vi "Scan.vi"(7 "Cluster":T1, 8 "Error":refnum<vi>, 9 "EMERGENCY":refnum<vi>, 10 "Scan in Progress":refnum<vi>, 11 "QUIT":refnum<vi>) -> ()   [LabVIEW 2018]
uses:
  <vilib>/Utility/file.llb/Write To Spreadsheet File (string).vi
  <vilib>/Utility/file.llb/Read From Spreadsheet File (string).vi
panel:
  out "Set VB?":bool
  out "Set VA?":bool
  out "Set VB":refnum<vi>
  out "Set VA":refnum<vi>
  out "Voltage Supply A":refnum<vi>
  out "Voltage Supply B":refnum<vi>
  out "Total Actions":i32
  out "GM1 ULD":refnum<vi>
  out "GM2 ULD":refnum<vi>
  out "GM2 LLD":refnum<vi>
  out "GM1 LLD":refnum<vi>
  out "Observables":string[][](array[string])
  out "GM2 Dwell":refnum<vi>
  out "GM1 Dwell":refnum<vi>
  out "Measure GM2":refnum<vi>
  out "GM2 Counts":refnum<vi>
  out "Measure GM1":refnum<vi>
  out "GM1 Counts":refnum<vi>
  out "ABORT":bool
  out "6487 Samples/measurement":refnum<vi>
  out "6485 Samples/measurement":refnum<vi>
  out "Theta Go":refnum<vi>
  out "Run All":bool
  out "X (mm)":refnum<vi>
  out "Y (mm)":refnum<vi>
  out "Z (mm)":refnum<vi>
  out "Theta (deg)":refnum<vi>
  out "Keithley6485 Current (A)":refnum<vi>
  out "Keithley6487 Current (A)":refnum<vi>
  out "Measure 6487":refnum<vi>
  out "Measure 6485":refnum<vi>
  out "Motors Are Active":refnum<vi>
  out "Set Motors":refnum<vi>
  out "Set EG":refnum<vi>
  out "Keithley6487 Potential (V)":refnum<vi>
  out "EG Y2 Alignment (V)":refnum<vi>
  out "EG Y1 Alignment (V)":refnum<vi>
  out "EG X2 Alignment (V)":refnum<vi>
  out "EG X1 Alignment (V)":refnum<vi>
  out "EG Filament (V)":refnum<vi>
  out "EG Focus 2 (V)":refnum<vi>
  out "EG Focus 1 (V)":refnum<vi>
  out "EG Extraction (V)":refnum<vi>
  out "EG Energy (eV)":refnum<vi>
  out "EG Grid (V)":refnum<vi>
  out "Set EG?":bool
  out "Theta Go To (mm)":refnum<vi>
  out "Z Go":refnum<vi>
  out "Z Go To (mm)":refnum<vi>
  out "Y Go":refnum<vi>
  out "Y Go To (mm)":refnum<vi>
  out "X Go To (mm)":refnum<vi>
  out "X Go":refnum<vi>
  out "Set Motors?":bool
  out "Current Task":string[](array[string])
  in  "Tasks":string[][](array[string])
  out "Independent Variables":string[][](array[string])
  in  "Scan.vi":enum32{"Scan", "Settings"}(tab)
  in  "Load Scan":bool
  in  "Generate Scan":bool
  in  "Dummy":dbl
  in  "Stop Scan":bool
  out "Status":string
  in  "Start Counting From...":i32
  out "Current File":path
  in  "Pending Tasks":i32(listbox)
  in  "Delete Task":bool
  in  "Clear Queue":bool
  out "Current Scan":string
  out "Current Action":string caption="Next Action"
  in  "Run All Scans":bool
  in  "Run One Scan":bool
  in  "Measurements":i32[](listbox)=[0]
  in  "Add to Queue":bool
  in  "Step Size":dbl=2.0 min=0.0 format="%#_4g"
  in  "End":dbl=11.0 format="%#_4g"
  in  "Start":dbl=1.0 format="%#_4g"
  in  "Variable":u16(ring) items=["X (mm)", "Y (mm)", "Z (mm)", "Theta (deg)", "EG Grid (V)", "EG Energy (eV)", "EG Extraction (V)", "EG Focus 1 (V)", "EG Focus 2 (V)", "EG Filament (V)", "EG X1 Alignment (V)", "EG X2 Alignment (V)", "EG Y1 Alignment (V)", "EG Y2 Alignment (V)", "6485 Samples", "6487 Samples", "6487 Voltage (V)", "GM2 Dwell Time (s)", "GM2 SCA Lower Limit (V)", "GM2 SCA Upper Limit (V)", "GM1 Dwell Time (s)", "GM1 SCA Lower Limit (V)", "GM1 SCA Upper Limit (V)", "Voltage Supply A", "Voltage Supply B", "Dummy"]
  in  "Folder":path=path "C:/data" caption="Save Directory"
  in  "Output Filename":string="Scan"
  in  "Scan File":path=path "C:/LabView VIs/IPES Scan Generator/Complex_Scan.scan"
  out "Progress:":i32
  in  "Settling time (ms)":u32
  in  "Output File Extension":string="dat"
  in  "Spacer in Output Filenames":string="_"
  in  "Number of Digits in Output Filename Suffix":i32=2
  in  "Character That Separates Parameters in Scan Commands":string=";"
  out "Observables Old":string[](array[string])
  # "%"
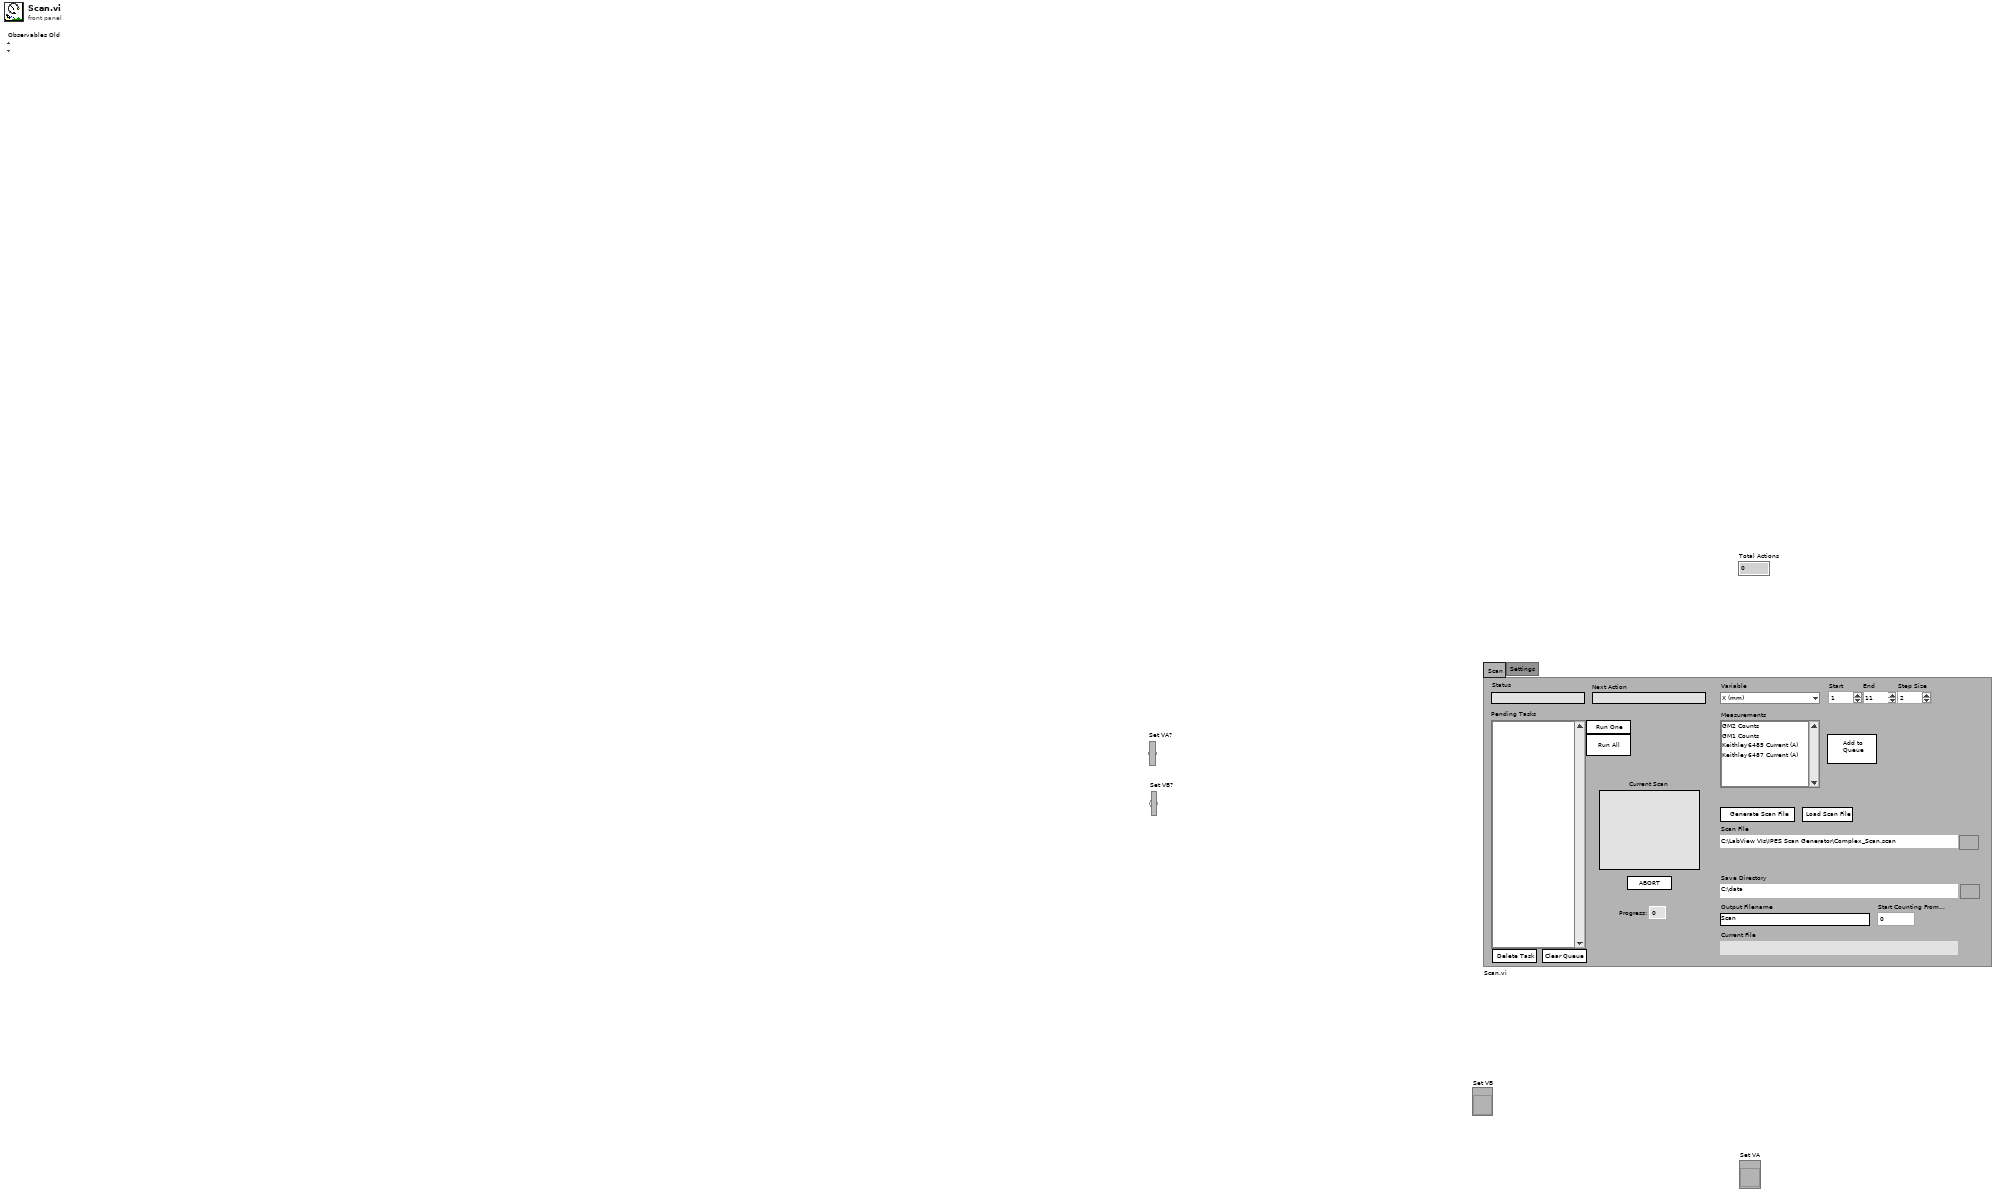
[diagram p1: front panel]
types:
  T1 = cluster{"EG Grid (V)":refnum<vi>, "EG Energy (eV)":refnum<vi>, "EG Extraction (V)":refnum<vi>, "EG Filament (V)":refnum<vi>, "EG Focus 1 (V)":refnum<vi>, "EG Focus 2 (V)":refnum<vi>, "EG X1 Alignment (V)":refnum<vi>, "EG X2 Alignment (V)":refnum<vi>, "EG Y1 Alignment (V)":refnum<vi>, "EG Y2 Alignment (V)":refnum<vi>, "Set EG":refnum<vi>, "X Go":refnum<vi>, "Y Go":refnum<vi>, "Z Go":refnum<vi>, "Theta Go":refnum<vi>, "X (mm)":refnum<vi>, "Y (mm)":refnum<vi>, "Z (mm)":refnum<vi>, "Theta (deg)":refnum<vi>, "X Go To (mm)":refnum<vi>, "Y Go To (mm)":refnum<vi>, "Z Go To (mm)":refnum<vi>, "Theta Go To (deg)":refnum<vi>, "Set Motors":refnum<vi>, "Motors Are Active":refnum<vi>, "Measure 6485":refnum<vi>, "Keithley6485 Current (A)":refnum<vi>, "6485 Samples/measurement":refnum<vi>, "Measure 6487":refnum<vi>, "Keithley6487 Current (A)":refnum<vi>, "Keithley6487 Voltage (V)":refnum<vi>, "6487 Samples/measurement":refnum<vi>, "GM Dwell Right":refnum<vi>, "GM LLD Right":refnum<vi>, "GM ULD Right":refnum<vi>, "GM Counts Right":refnum<vi>, "Measure GM Right":refnum<vi>, "GM Dwell Left":refnum<vi>, "GM LLD Left":refnum<vi>, "GM ULD Left":refnum<vi>, "GM Counts Left":refnum<vi>, "Measure GM Left":refnum<vi>, "Voltage Supply B":refnum<vi>, "Voltage Supply A":refnum<vi>, "Set VA":refnum<vi>, "Set VB":refnum<vi>}
  T2 = enum16{"open", "replace", "create", "open or create", "replace or create", "replace or create with confirmation"}
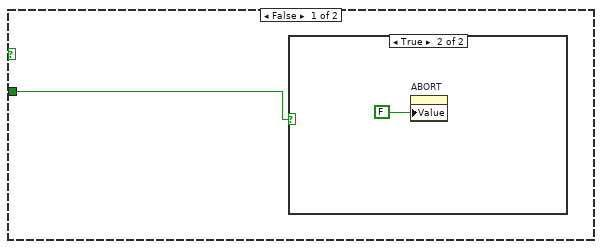
[diagram p14: hidden frame]
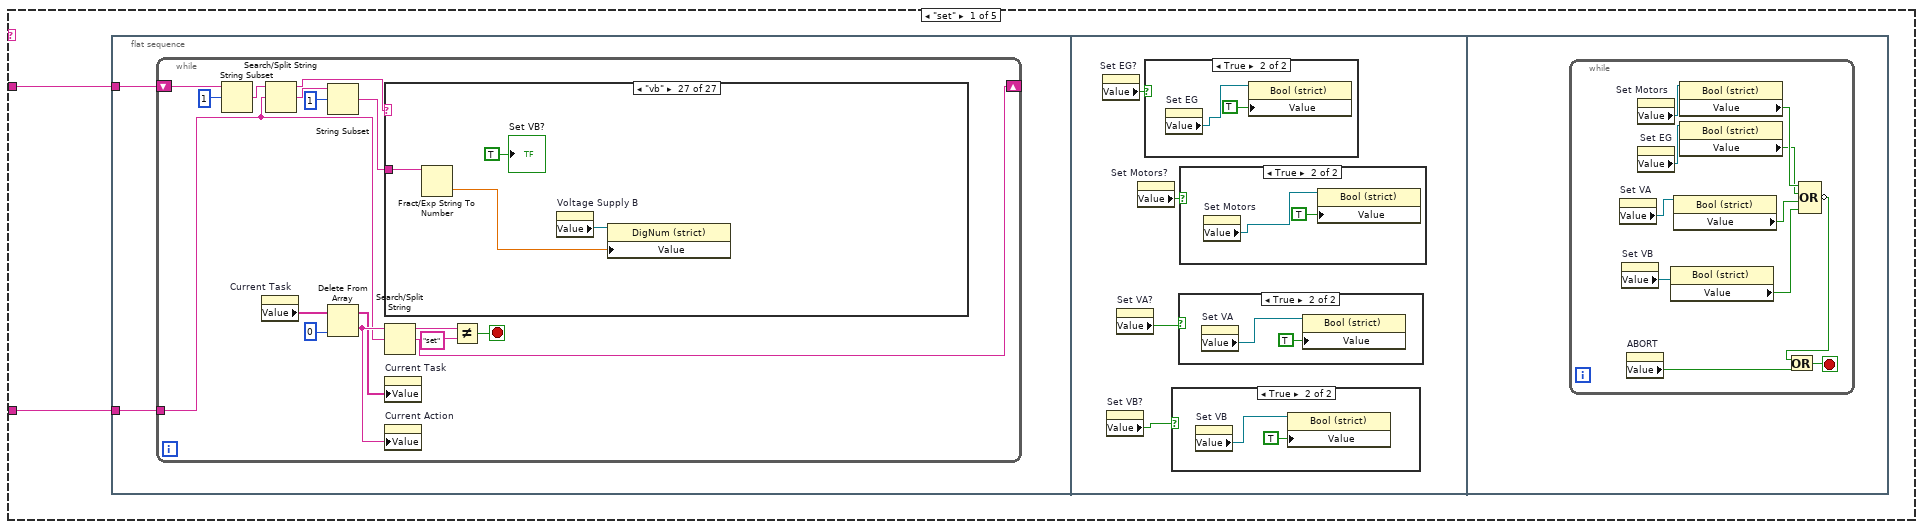
[diagram p17: hidden frame]
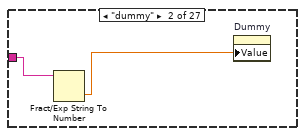
[diagram p19: hidden frame]
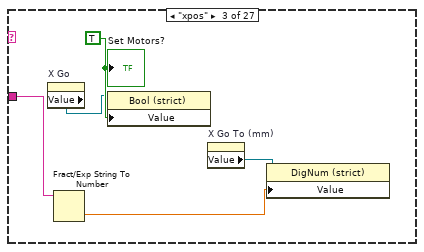
[diagram p20: hidden frame]
diagram:
  n1 = flat-sequence {
    frame #0 {
      w1 = FALSE ("Set Motors?")
      w2 = FALSE ("Visible")
      # "<Tasks> is a 2D list.  Every row represents a scan, and every element in a row is a scan command.  Note that rows can have different lengths.  When a scan is executed, it is popped off the top of <Tasks> and then its commands are executed in order.\n\n<Pending Tasks> is the 1D list of scans that the user sees.  Every element represents a scan and contains the meta data shown on the front panel."
      # "Initialization, variable declaration, etc..."
      n2 = Unbundle("Cluster") -> ("EG Grid (V)"=→"EG Grid (V)":refnum<vi>, "EG Energy (eV)"=→"EG Energy (eV)":refnum<vi>, "EG Extraction (V)"=→"EG Extraction (V)":refnum<vi>, "EG Filament (V)"=→"EG Filament (V)":refnum<vi>, "EG Focus 1 (V)"=→"EG Focus 1 (V)":refnum<vi>, "EG Focus 2 (V)"=→"EG Focus 2 (V)":refnum<vi>, "EG X1 Alignment (V)"=→"EG X1 Alignment (V)":refnum<vi>, "EG X2 Alignment (V)"=→"EG X2 Alignment (V)":refnum<vi>, "EG Y1 Alignment (V)"=→"EG Y1 Alignment (V)":refnum<vi>, "EG Y2 Alignment (V)"=→"EG Y2 Alignment (V)":refnum<vi>, "Set EG"=→"Set EG":refnum<vi>, "X Go"=→"X Go":refnum<vi>, "Y Go"=→"Y Go":refnum<vi>, "Z Go"=→"Z Go":refnum<vi>, "Theta Go"=→"Theta Go":refnum<vi>, "X (mm)"=→"X (mm)":refnum<vi>, "Y (mm)"=→"Y (mm)":refnum<vi>, "Z (mm)"=→"Z (mm)":refnum<vi>, "Theta (deg)"=→"Theta (deg)":refnum<vi>, "X Go To (mm)"=→"X Go To (mm)":refnum<vi>, "Y Go To (mm)"=→"Y Go To (mm)":refnum<vi>, "Z Go To (mm)"=→"Z Go To (mm)":refnum<vi>, "Theta Go To (deg)"=→"Theta Go To (mm)":refnum<vi>, "Set Motors"=→"Set Motors":refnum<vi>, "Motors Are Active"=→"Motors Are Active":refnum<vi>, "Measure 6485"=→"Measure 6485":refnum<vi>, "Keithley6485 Current (A)"=→"Keithley6485 Current (A)":refnum<vi>, "6485 Samples/measurement"=→"6485 Samples/measurement":refnum<vi>, "Measure 6487"=→"Measure 6487":refnum<vi>, "Keithley6487 Current (A)"=→"Keithley6487 Current (A)":refnum<vi>, "Keithley6487 Voltage (V)"=→"Keithley6487 Potential (V)":refnum<vi>, "6487 Samples/measurement"=→"6487 Samples/measurement":refnum<vi>, "GM Dwell Right"=→"GM1 Dwell":refnum<vi>, "GM LLD Right"=→"GM1 LLD":refnum<vi>, "GM ULD Right"=→"GM1 ULD":refnum<vi>, "GM Counts Right"=→"GM1 Counts":refnum<vi>, "Measure GM Right"=→"Measure GM1":refnum<vi>, "GM Dwell Left"=→"GM2 Dwell":refnum<vi>, "GM LLD Left"=→"GM2 LLD":refnum<vi>, "GM ULD Left"=→"GM2 ULD":refnum<vi>, "GM Counts Left"=→"GM2 Counts":refnum<vi>, "Measure GM Left"=→"Measure GM2":refnum<vi>, "Voltage Supply B"=→"Voltage Supply B":refnum<vi>, "Voltage Supply A"=→"Voltage Supply A":refnum<vi>, "Set VA"=→"Set VA":refnum<vi>, "Set VB"=→"Set VB":refnum<vi>)
      n3 = Initialize Array("", 0 ("dimension size")) -> (→"Current Task":string[])
      n4 = Build Array("gm2" ("element"), "gm1" ("element"), "6485c", "6487c") -> (w57:string[])
      n5 = Delete From Array(array="Tasks", index (col)=0 ("disabled index (col)")) -> (deleted portion=w117:string[])  [unwired: 2 in, 1 out]
      n6 = property on="Set VB?" class="Bool (strict)"("Value"=w1) -> ()  [unwired: 2 in, 2 out]
      n7 = property on="Set EG?" class="Bool (strict)"("Value"=w1) -> ()  [unwired: 2 in, 2 out]
      n8 = property on="Set Motors?" class="Bool (strict)"("Value"=w1) -> ()  [unwired: 2 in, 2 out]
      n9 = property on="Set VA?" class="Bool (strict)"("Value"=w1) -> ()  [unwired: 2 in, 2 out]
      n10 = property on="Pending Tasks" class="LstBox (strict)"("Item Names"=w117) -> ()  [unwired: 2 in, 2 out]
      n11 = Build Array("GM2 Counts" ("element"), "GM1 Counts" ("element"), "Keithley6485 Current (A)", "Keithley6487 Current (A)") -> (w58:string[])
      n12 = Build Array(w58, w57) -> (→"Observables":string[][])
      n13 = property on="Measurements" class="LstBox (strict)"("Item Names"=w58) -> ()  [unwired: 2 in, 2 out]
      n14 = Build Array("xpos", "ypos", "zpos", "theta", "grid", "en", "ext", "f1", "f2", "fil", "x1", "x2", "y1", "y2", "6485s", "6487s", "6487v", "gm2dw" ("element"), "gm2ll" ("element"), "gm2ul" ("element"), "gm1dw" ("element"), "gm1ll" ("element"), "gm1ul" ("element"), "va" ("element"), "vb" ("element"), "dummy" ("element")) -> (w116:string[])
      n15 = Build Array("X (mm)", "Y (mm)", "Z (mm)", "Theta (deg)", "EG Grid (V)", "EG Energy (eV)", "EG Extraction (V)", "EG Focus 1 (V)", "EG Focus 2 (V)", "EG Filament (V)", "EG X1 Alignment (V)", "EG X2 Alignment (V)", "EG Y1 Alignment (V)", "EG Y2 Alignment (V)", "6485 Samples", "6487 Samples", "6487 Voltage (V)", "GM2 Dwell Time (s)" ("element"), "GM2 SCA Lower Limit (V)" ("element"), "GM2 SCA Upper Limit (V)" ("element"), "GM1 Dwell Time (s)" ("element"), "GM1 SCA Lower Limit (V)" ("element"), "GM1 SCA Upper Limit (V)" ("element"), "Voltage Supply A (V)" ("element"), "Voltage Supply B (V)" ("element"), "Dummy" ("element")) -> (w59:string[])
      n16 = Build Array(w59, w116) -> (→"Independent Variables":string[][])
      n17 = property on="Variable" class="Ring (strict)"("Strings []"=w59) -> ()  [unwired: 2 in, 2 out]
      n18 = property on="Set Motors" class="LVObjRef (strict)"("Visible"=w2) -> ()  [unwired: 2 in, 2 out]
      n19 = property on="X Go To (mm)" class="LVObjRef (strict)"("Visible"=w2) -> ()  [unwired: 2 in, 2 out]
      n20 = property on="Set EG" class="LVObjRef (strict)"("Visible"=w2) -> ()  [unwired: 2 in, 2 out]
      n21 = property on="Z Go" class="LVObjRef (strict)"("Visible"=w2) -> ()  [unwired: 2 in, 2 out]
      n22 = property on="Y Go" class="LVObjRef (strict)"("Visible"=w2) -> ()  [unwired: 2 in, 2 out]
      n23 = property on="X Go" class="LVObjRef (strict)"("Visible"=w2) -> ()  [unwired: 2 in, 2 out]
      n24 = property on="Set Motors?" class="Bool (strict)"("Visible"=w2) -> ()  [unwired: 2 in, 2 out]
      n25 = property on="EG Grid (V)" class="LVObjRef (strict)"("Visible"=w2) -> ()  [unwired: 2 in, 2 out]
      n26 = property on="EG Focus 1 (V)" class="LVObjRef (strict)"("Visible"=w2) -> ()  [unwired: 2 in, 2 out]
      n27 = property on="EG Focus 2 (V)" class="LVObjRef (strict)"("Visible"=w2) -> ()  [unwired: 2 in, 2 out]
      n28 = property on="Z Go To (mm)" class="LVObjRef (strict)"("Visible"=w2) -> ()  [unwired: 2 in, 2 out]
      n29 = property on="QUIT" class="LVObjRef (strict)"("Visible"=w2) -> ()  [unwired: 2 in, 2 out]
      n30 = property on="Y Go To (mm)" class="LVObjRef (strict)"("Visible"=w2) -> ()  [unwired: 2 in, 2 out]
      n31 = property on="X (mm)" class="LVObjRef (strict)"("Visible"=w2) -> ()  [unwired: 2 in, 2 out]
      n32 = property on="ABORT" class="Bool (strict)"("Visible"=w2) -> ()  [unwired: 2 in, 2 out]
      n33 = property on="Theta (deg)" class="LVObjRef (strict)"("Visible"=w2) -> ()  [unwired: 2 in, 2 out]
      n34 = property on="Theta Go" class="LVObjRef (strict)"("Visible"=w2) -> ()  [unwired: 2 in, 2 out]
      n35 = property on="Run All" class="Bool (strict)"("Visible"=w2) -> ()  [unwired: 2 in, 2 out]
      n36 = property on="Z (mm)" class="LVObjRef (strict)"("Visible"=w2) -> ()  [unwired: 2 in, 2 out]
      n37 = property on="Y (mm)" class="LVObjRef (strict)"("Visible"=w2) -> ()  [unwired: 2 in, 2 out]
      n38 = property on="Set EG?" class="Bool (strict)"("Visible"=w2) -> ()  [unwired: 2 in, 2 out]
      n39 = property on="Error" class="LVObjRef (strict)"("Visible"=w2) -> ()  [unwired: 2 in, 2 out]
      n40 = property on="Measure 6487" class="LVObjRef (strict)"("Visible"=w2) -> ()  [unwired: 2 in, 2 out]
      n41 = property on="EMERGENCY" class="LVObjRef (strict)"("Visible"=w2) -> ()  [unwired: 2 in, 2 out]
      n42 = property on="Measure 6485" class="LVObjRef (strict)"("Visible"=w2) -> ()  [unwired: 2 in, 2 out]
      n43 = property on="Dummy" class="DigNum (strict)"("Visible"=w2) -> ()  [unwired: 2 in, 2 out]
      n44 = property on="Current Task" class="Arr (strict)"("Visible"=w2) -> ()  [unwired: 2 in, 2 out]
      n45 = property on="Tasks" class="Arr (strict)"("Visible"=w2) -> ()  [unwired: 2 in, 2 out]
      n46 = property on="EG Y2 Alignment (V)" class="LVObjRef (strict)"("Visible"=w2) -> ()  [unwired: 2 in, 2 out]
      n47 = property on="Keithley6487 Potential (V)" class="LVObjRef (strict)"("Visible"=w2) -> ()  [unwired: 2 in, 2 out]
      n48 = property on="EG Filament (V)" class="LVObjRef (strict)"("Visible"=w2) -> ()  [unwired: 2 in, 2 out]
      n49 = property on="Theta Go To (mm)" class="LVObjRef (strict)"("Visible"=w2) -> ()  [unwired: 2 in, 2 out]
      n50 = property on="Independent Variables" class="Arr (strict)"("Visible"=w2) -> ()  [unwired: 2 in, 2 out]
      n51 = property on="EG X1 Alignment (V)" class="LVObjRef (strict)"("Visible"=w2) -> ()  [unwired: 2 in, 2 out]
      n52 = property on="EG Extraction (V)" class="LVObjRef (strict)"("Visible"=w2) -> ()  [unwired: 2 in, 2 out]
      n53 = property on="EG X2 Alignment (V)" class="LVObjRef (strict)"("Visible"=w2) -> ()  [unwired: 2 in, 2 out]
      n54 = property on="EG Energy (eV)" class="LVObjRef (strict)"("Visible"=w2) -> ()  [unwired: 2 in, 2 out]
      n55 = property on="EG Y1 Alignment (V)" class="LVObjRef (strict)"("Visible"=w2) -> ()  [unwired: 2 in, 2 out]
      n56 = property on="Motors Are Active" class="LVObjRef (strict)"("Visible"=w2) -> ()  [unwired: 2 in, 2 out]
      n57 = property on="6485 Samples/measurement" class="LVObjRef (strict)"("Visible"=w2) -> ()  [unwired: 2 in, 2 out]
      n58 = property on="Keithley6485 Current (A)" class="LVObjRef (strict)"("Visible"=w2) -> ()  [unwired: 2 in, 2 out]
      n59 = property on="Keithley6487 Current (A)" class="LVObjRef (strict)"("Visible"=w2) -> ()  [unwired: 2 in, 2 out]
      n60 = property on="Scan in Progress" class="LVObjRef (strict)"("Visible"=w2) -> ()  [unwired: 2 in, 2 out]
      n61 = property on="GM1 Counts" class="LVObjRef (strict)"("Visible"=w2) -> ()  [unwired: 2 in, 2 out]
      n62 = property on="Measure GM1" class="LVObjRef (strict)"("Visible"=w2) -> ()  [unwired: 2 in, 2 out]
      n63 = property on="Measure GM2" class="LVObjRef (strict)"("Visible"=w2) -> ()  [unwired: 2 in, 2 out]
      n64 = property on="GM2 Counts" class="LVObjRef (strict)"("Visible"=w2) -> ()  [unwired: 2 in, 2 out]
      n65 = property on="EG Y2 Alignment (V)" class="LVObjRef (strict)"("Visible"=w2) -> ()  [unwired: 2 in, 2 out]
      n66 = property on="GM1 Dwell" class="LVObjRef (strict)"("Visible"=w2) -> ()  [unwired: 2 in, 2 out]
      n67 = property on="Voltage Supply A" class="LVObjRef (strict)"("Visible"=w2) -> ()  [unwired: 2 in, 2 out]
      n68 = property on="6487 Samples/measurement" class="LVObjRef (strict)"("Visible"=w2) -> ()  [unwired: 2 in, 2 out]
      n69 = property on="GM2 Dwell" class="LVObjRef (strict)"("Visible"=w2) -> ()  [unwired: 2 in, 2 out]
      n70 = property on="GM1 LLD" class="LVObjRef (strict)"("Visible"=w2) -> ()  [unwired: 2 in, 2 out]
      n71 = property on="GM2 LLD" class="LVObjRef (strict)"("Visible"=w2) -> ()  [unwired: 2 in, 2 out]
      n72 = property on="Observables" class="Arr (strict)"("Visible"=w2) -> ()  [unwired: 2 in, 2 out]
      n73 = property on="GM2 ULD" class="LVObjRef (strict)"("Visible"=w2) -> ()  [unwired: 2 in, 2 out]
      n74 = property on="GM1 ULD" class="LVObjRef (strict)"("Visible"=w2) -> ()  [unwired: 2 in, 2 out]
      n75 = property on="Voltage Supply B" class="LVObjRef (strict)"("Visible"=w2) -> ()  [unwired: 2 in, 2 out]
      n76 = property on="Cluster" class="Clust (strict)"("Visible"=w2) -> ()  [unwired: 2 in, 2 out]
      "ABORT" <- FALSE ("ABORT")
    }
    frame #1 {
      n77 = while {
        stop <- w131 stop-if-true
        # "This loops deals with all the buttons, etc., for the user interface.  Constantly checking to see if a button has been pushed.  If it has, execute some action."
        n78 = property class="Bool (strict)"(reference="EMERGENCY") -> ("Value"=w126:bool)  [unwired: 1 in, 2 out]
        n79 = case shown="True" "Add to Queue" {
          frame False {
          }
          frame True {
            w264 = "\r\n"
            w280 = "%#g" ("format string")
            # "Generate the 1D scan and add it to <Tasks> and <Pending Tasks>."
            n80 = property on="Character That Separates Parameters in Scan Commands" class="Str"() -> ("Value"=w266:string)  [unwired: 2 in, 2 out]
            n81 = Initialize Array("", 0 ("dimension size")) -> (w297:string[])
            n82 = Array Size(array="Measurements") -> (size(s)=w300:i32)
            n83 = for {
              N: w300 -> [_]
              tunnel: "Measurements" -> [w326]
              tunnel: w266 -> [w312]
              shift-right: [w322] -> w296
              shift-left: w297 -> [w325]
              shift-right: [w320] -> w277
              shift-left: "" -> [w321]
              i -> [w317]
              n84 = property on="Observables" class="Arr (strict)"() -> ("Value"=w315:string[][])  [unwired: 2 in, 2 out]
              n85 = Equal To 0?(x=w317) -> (x = 0?=w316:bool)
              n86 = Index Array(array=w326, index=w317) -> (element=w314:i32)
              n87 = case shown="False" w316 {
                tunnel: [", " _] -> w319
                frame False {
                }
                frame True {
                }
              }
              n88 = Index Array(array=w315, index (row)=1 ("disabled index (row)"), index (col)=w314) -> (element=w318:string)
              n89 = Concatenate Strings("measure", w312, w318, w312) -> (w323:string)
              n90 = Concatenate Strings(w321, w319, w318) -> (w320:string)
              n91 = Build Array (concatenate)(w325, w323) -> (w322:string[])
            }
            n92 = Subtract(x="End", y="Start") -> (x-y=w310:dbl)
            n93 = Greater?(x="Start", y="End") -> (0:w303:bool)
            n94 = case shown="True" w303 {
              tunnel: "Step Size" -> [w328 w330]
              tunnel: [w328 w329] -> w302
              frame False {
              }
              frame True {
                n95 = Negate(x=w330) -> (-x=w329:dbl)
              }
            }
            n96 = Divide(x=w310, y="Step Size") -> (x/y=w305:dbl)
            n97 = property on="Independent Variables" class="Arr (strict)"() -> ("Value"=w276:string[][])  [unwired: 2 in, 2 out]
            n98 = Absolute Value(x=w305) -> (abs(x)=w304:dbl)
            n99 = Increment(x=w304) -> (x+1=w311:dbl)
            n100 = Round Toward -Infinity(1:w311) -> (0:w270:dbl)
            n101 = Index Array(array=w276, index (row)=0 ("disabled index (col)"), index (col)="Variable") -> (element=w309:string)
            n102 = Index Array(array=w276, index (row)=1 ("disabled index (col)"), index (col)="Variable") -> (element=w301:string)
            n103 = Initialize Array("", 0 ("dimension size")) -> (w292:string[])
            n104 = Format Value(format string=w280, value (0)="Start") -> (output string=w286:string)  [unwired: 1 in]
            n105 = Format Value(format string=w280, value (0)="Step Size") -> (output string=w283:string)  [unwired: 1 in]
            n106 = Format Value(format string=w280, value (0)="End") -> (output string=w281:string)  [unwired: 1 in]
            n107 = for {
              N: w270 -> [_]
              tunnel: w302 -> [w339]
              tunnel: "Start" -> [w341]
              tunnel: w266 -> [w331]
              tunnel: w301 -> [w342]
              tunnel: w296 -> [w334]
              shift-right: [w333] -> w295
              shift-left: w292 -> [w332]
              i -> [w338]
              n108 = Multiply(x=w339, y=w338) -> (x*y=w340:dbl)
              n109 = Add(x=w341, y=w340) -> (x+y=w337:dbl)
              n110 = Number To Fractional String(number=w337) -> (F-format string=w336:string)  [unwired: 3 in]
              n111 = Concatenate Strings("set" ("string"), w331, w342, w331, w336, w331) -> (w335:string)
              n112 = Build Array (concatenate)(w332, w335, w334) -> (w333:string[])
            }
            n113 = property on="Pending Tasks" class="LstBox (strict)"() -> ("Item Names"=w274:string[])  [unwired: 2 in, 2 out]
            n114 = Number To Decimal String(number=w270) -> (decimal integer string=w269:string)  [unwired: 1 in]
            n115 = Concatenate Strings(w309, w264, "From ", w286, " To ", w281, " By ", w283, w264, "Measure " ("string"), w277, w264, w269, " points" ("string")) -> (w290:string)
            n116 = Build Array (concatenate)(w274, w290) -> (w273:string[])
            n117 = property on="Pending Tasks" class="LstBox (strict)"("Item Names"=w273) -> ()  [unwired: 2 in, 2 out]
            n118 = Concatenate Strings("end" ("element"), w266) -> (w265:string)
            n119 = Build Array (concatenate)(w290, w295, w265) -> (w291:string[])
            n120 = property on="Tasks" class="Arr (strict)"() -> ("Value"=w272:string[][])  [unwired: 2 in, 2 out]
            n121 = Build Array (concatenate)(w272, w291) -> (w271:string[][])
            n122 = property on="Tasks" class="Arr (strict)"("Value"=w271) -> ()  [unwired: 2 in, 2 out]
          }
        }
        n123 = case shown="True" "Stop Scan" {
          frame False {
          }
          frame True {
            # "Abort current scan and don't run the next one (if any are queued)."
            n124 = call <vilib>:"Beep.vi"("use system alert? (T)"=FALSE, "duration (msec)"=u32 300 ("frequency (Hz)"), "frequency (Hz)"=u32 250 ("duration (msec)")) -> ()  [unwired: 9 in]
            n125 = property on="Run All" class="Bool (strict)"("Value"=FALSE ("Run All")) -> ()  [unwired: 2 in, 2 out]
            n126 = property on="Current Action" class="Str"("Value"="") -> ()  [unwired: 2 in, 2 out]
            n127 = property on="ABORT" class="Bool (strict)"("Value"=TRUE ("ABORT")) -> ()  [unwired: 2 in, 2 out]
            n128 = property on="Current Scan" class="Str"() -> ("Value"=w246:string)  [unwired: 2 in, 2 out]
            n129 = Initialize Array("", 0 ("dimension size")) -> (w241:string[])
            n130 = property on="Current Task" class="Arr (strict)"("Value"=w241) -> ()  [unwired: 2 in, 2 out]
            n131 = Concatenate Strings("~Aborted~\n" ("string"), w246) -> (w244:string)
            n132 = property on="Scan in Progress" class="LVObjRef (strict)"() -> ("Value"=w249:refnum<vi>)  [unwired: 2 in, 2 out]
            n133 = property on="Current Scan" class="Str"("Value"=w244) -> ()  [unwired: 2 in, 2 out]
            n134 = property on="Status" class="Str"("Value"="Aborting Scan" ("Status")) -> ()  [unwired: 2 in, 2 out]
            n135 = property class="Bool (strict)"(reference=w249, "Value"=FALSE) -> ()  [unwired: 1 in, 2 out]
          }
        }
        n136 = case shown="True" "Clear Queue" {
          frame False {
          }
          frame True {
            # "Remove all scans from the list of scans."
            n137 = Initialize Array("", 0 ("dimension size"), 0 ("dimension size")) -> (w253:string[][])
            n138 = Initialize Array("", 0) -> (w252:string[])
            n139 = property on="Tasks" class="Arr (strict)"("Value"=w253) -> ()  [unwired: 2 in, 2 out]
            n140 = property on="Pending Tasks" class="LstBox (strict)"("Item Names"=w252) -> ()  [unwired: 2 in, 2 out]
          }
        }
        n141 = case shown="True" "Delete Task" {
          frame False {
          }
          frame True {
            # "Remove the selected scan from the list of scans."
            n142 = property on="Pending Tasks" class="LstBox (strict)"() -> ("Item Names"=w263:string[])  [unwired: 2 in, 2 out]
            n143 = property on="Tasks" class="Arr (strict)"() -> ("Value"=w260:string[][])  [unwired: 2 in, 2 out]
            n144 = Delete From Array(array=w263, index="Pending Tasks") -> (array with subset deleted=w262:string[])  [unwired: 1 in, 1 out]
            n145 = property on="Pending Tasks" class="LstBox (strict)"("Item Names"=w262) -> ()  [unwired: 2 in, 2 out]
            n146 = Delete From Array(array=w260, index (row)="Pending Tasks") -> (array with subset deleted=w259:string[][])  [unwired: 2 in, 1 out]
            n147 = property on="Tasks" class="Arr (strict)"("Value"=w259) -> ()  [unwired: 2 in, 2 out]
          }
        }
        n148 = case shown="True" w126 {
          frame False {
          }
          frame True {
            # "Stop all scans."
            n149 = property on="ABORT" class="Bool (strict)"("Value"=TRUE ("ABORT")) -> ()  [unwired: 2 in, 2 out]
          }
        }
        n150 = property on="QUIT" class="LVObjRef (strict)"() -> ("Value"=w132:refnum<vi>)  [unwired: 2 in, 2 out]
        n151 = property class="Bool (strict)"(reference=w132) -> ("Value"=w131:bool)  [unwired: 1 in, 2 out]
        n152 = case shown="True" "Generate Scan" {
          frame False {
          }
          frame True {
            w204 = "\"" ("string")
            # "Execute the external scan generating application using OS functions.  Collect various information from the <settings.conf> configuration file."
            n153 = Current VI's Path() -> (path=w211:path)
            n154 = Current VI's Path() -> (path=w192:path)
            n155 = Strip Path(path=w211) -> (stripped path=w207:path)  [unwired: 1 out]
            n156 = Strip Path(path=w192) -> (stripped path=w196:path)  [unwired: 1 out]
            n157 = Strip Path(path=w207) -> (stripped path=w206:path)  [unwired: 1 out]
            n158 = Strip Path(path=w196) -> (stripped path=w197:path)  [unwired: 1 out]
            n159 = Build Path(base path=w206, name or relative path="IPES Scan Generator") -> (appended path=w209:path)
            n160 = Build Path(base path=w197, name or relative path="IPES Scan Generator") -> (appended path=w194:path)
            n161 = Path To String(path=w209) -> (string=w208:string)
            n162 = Path To String(path=w194) -> (string=w195:string)
            n163 = Concatenate Strings(w195, "\\src\\settings.conf" ("string")) -> (w191:string)
            n164 = String To Path(string=w191) -> (path=w190:path)
            n165 = Concatenate Strings("C:\\Python32\\python.exe " ("command line"), w204, w208, "/src/jener8or.py" ("string"), w204) -> (w202:string)
            n166 = Read from Text File(file (use dialog)=w190) -> (text=w175:string)  [unwired: 3 in, 3 out]
            n167 = while {
              tunnel: [w232] -> w200 mode=indexing
              tunnel: "[Pp][Aa][Tt][Hh][\\s\\t]+=[\\s\\t]+" ("search string") -> [w230]
              shift-right: [w229] -> _
              shift-left: w175 -> [w231]
              stop <- w228 stop-if-true
              n168 = Match Pattern(string=w231, regular expression=w230) -> (after substring=w233:string)  [unwired: 1 in, 3 out]
              n169 = Match Pattern(string=w233, regular expression="[\\n]") -> (before substring=w232:string, after substring=w229:string)  [unwired: 1 in, 2 out]
              n170 = Equal?(x=w232, y="") -> (x = y?=w228:bool)
            }
            n171 = call <vilib>:"System Exec.vi"("wait until completion? (T)"=FALSE, "command line"=w202) -> ()  [unwired: 6 in, 4 out]
            n172 = while {
              tunnel: [w224] -> w182 mode=indexing
              tunnel: "[Ff][Ii][Ll][Ee][Nn][Aa][Mm][Ee][\\s\\t]+=[\\s\\t]+" ("search string") -> [w222]
              shift-right: [w221] -> _
              shift-left: w175 -> [w223]
              stop <- w220 stop-if-true
              n173 = Match Pattern(string=w223, regular expression=w222) -> (after substring=w225:string)  [unwired: 1 in, 3 out]
              n174 = Match Pattern(string=w225, regular expression="[\\n]") -> (before substring=w224:string, after substring=w221:string)  [unwired: 1 in, 2 out]
              n175 = Equal?(x=w224, y="") -> (x = y?=w220:bool)
            }
            n176 = while {
              tunnel: [w216] -> w179 mode=indexing
              tunnel: "[Ss][Ee][Pp][Aa][Rr][Aa][Tt][Oo][Rr][\\s\\t]+=[\\s\\t\\]+" ("search string") -> [w214]
              shift-right: [w213] -> _
              shift-left: w175 -> [w215]
              stop <- w212 stop-if-true
              n177 = Match Pattern(string=w215, regular expression=w214) -> (after substring=w217:string)  [unwired: 1 in, 3 out]
              n178 = Match Pattern(string=w217, regular expression="[\\n]") -> (before substring=w216:string, after substring=w213:string)  [unwired: 1 in, 2 out]
              n179 = Equal?(x=w216, y="") -> (x = y?=w212:bool)
            }
            n180 = Array Size(array=w200) -> (size(s)=w199:i32)
            n181 = Array Size(array=w182) -> (size(s)=w183:i32)
            n182 = Array Size(array=w179) -> (size(s)=w176:i32)
            n183 = Decrement(x=w199) -> (x-1=w188:i32)
            n184 = Decrement(x=w183) -> (x-1=w184:i32)
            n185 = Decrement(x=w176) -> (x-1=w177:i32)
            n186 = Decrement(x=w188) -> (x-1=w187:i32)
            n187 = Decrement(x=w184) -> (x-1=w185:i32)
            n188 = Decrement(x=w177) -> (x-1=w178:i32)
            n189 = Index Array(array=w200, index=w187) -> (element=w173:string)
            n190 = Index Array(array=w182, index=w185) -> ()  [unwired: 1 out]
            n191 = Index Array(array=w179, index=w178) -> (element=w181:string)
            n192 = property on="Character That Separates Parameters in Scan Commands" class="Str"("Value"=w181) -> ()  [unwired: 2 in, 2 out]
            n193 = String To Path(string=w173) -> (path=w174:path)
            n194 = property on="Scan File" class="Path"("Value"=w174) -> ()  [unwired: 2 in, 2 out]
          }
        }
        n195 = Or(x="Run One Scan", y="Run All Scans") -> (x .or. y?=w125:bool)
        n196 = case shown="True" w125 {
          tunnel: "Run All Scans" -> [_ w357]
          frame False {
          }
          frame True {
            # "Toggle the <Scan in Progress> flag on.  Turn all <Set #> and <Measure #> flags off.  If the user pressed \"Run All Scans,\" then turn the <Run All> flag on."
            n197 = property on="Run All" class="Bool (strict)"("Value"=w357) -> ()  [unwired: 2 in, 2 out]
            n198 = property on="Scan in Progress" class="LVObjRef (strict)"() -> ("Value"=w359:refnum<vi>)  [unwired: 2 in, 2 out]
            n199 = property class="Bool (strict)"(reference=w359, "Value"=TRUE ("Scan In Progress")) -> ()  [unwired: 1 in, 2 out]
            n200 = property on="Status" class="Str"("Value"="Initializing Scan\n(Getting Last Measurements)") -> ()  [unwired: 2 in, 2 out]
            n201 = property on="Set EG" class="LVObjRef (strict)"() -> ("Value"=w354:refnum<vi>)  [unwired: 2 in, 2 out]
            n202 = property on="Set Motors" class="LVObjRef (strict)"() -> ("Value"=w355:refnum<vi>)  [unwired: 2 in, 2 out]
            n203 = property class="Bool (strict)"(reference=w354, "Value"=FALSE) -> ()  [unwired: 1 in, 2 out]
            n204 = property class="Bool (strict)"(reference=w355, "Value"=FALSE) -> ()  [unwired: 1 in, 2 out]
            n205 = disable-structure shown="Disabled" {
              frame Disabled {
                n206 = property on="Measure GM2" class="LVObjRef (strict)"() -> ("Value"=w360:refnum<vi>)  [unwired: 2 in, 2 out]
                n207 = property class="Bool (strict)"(reference=w360, "Value"=TRUE) -> ()  [unwired: 1 in, 2 out]
              }
              frame Enabled {
              }
            }
            n208 = property on="Measure GM1" class="LVObjRef (strict)"() -> ("Value"=w351:refnum<vi>)  [unwired: 2 in, 2 out]
            n209 = property class="Bool (strict)"(reference=w351, "Value"=TRUE) -> ()  [unwired: 1 in, 2 out]
            n210 = property on="Measure 6485" class="LVObjRef (strict)"() -> ("Value"=w349:refnum<vi>)  [unwired: 2 in, 2 out]
            n211 = property on="Measure 6487" class="LVObjRef (strict)"() -> ("Value"=w346:refnum<vi>)  [unwired: 2 in, 2 out]
            n212 = property class="Bool (strict)"(reference=w349, "Value"=TRUE ("Measure 6485")) -> ()  [unwired: 1 in, 2 out]
            n213 = property class="Bool (strict)"(reference=w346, "Value"=TRUE ("Measure 6485")) -> ()  [unwired: 1 in, 2 out]
            n214 = property on="Set EG?" class="Bool (strict)"("Value"=FALSE ("Set EG?")) -> ()  [unwired: 2 in, 2 out]
            n215 = property on="Set Motors?" class="Bool (strict)"("Value"=FALSE ("Set Motors?")) -> ()  [unwired: 2 in, 2 out]
          }
        }
        n216 = case shown="True" "Load Scan" {
          frame False {
          }
          frame True {
            # "Load a scan from the specified file and add it to <Tasks>.  Add meta data to <Pending Tasks>."
            n217 = call-poly <vilib>:"Read From Spreadsheet File.vi"("file path (dialog if empty)"="Scan File") -> ("all rows"=w153:string[][])  [unwired: 6 in, 4 out]
            n218 = Index Array(array=w153, index (col)=0 ("disabled index (col)")) -> (element=w149:string[])  [unwired: 1 in]
            n219 = while {
              shift-right: [w158] -> _
              shift-left: w149 -> [w160]
              tunnel: [w159] -> w147 mode=indexing
              tunnel: [w158] -> w138
              stop <- w162 continue-if-true
              n220 = Delete From Array(array=w160, index=0) -> (deleted portion=w163:string, array with subset deleted=w161:string[])  [unwired: 1 in]
              n221 = String Subset(string=w163, length (rest)=1 ("length (rest)")) -> (substring=w165:string)  [unwired: 1 in]
              n222 = Equal?(x="#" ("search string"), y=w165) -> (x = y?=w162:bool)
              n223 = case shown="True" w162 {
                tunnel: w163 -> [_ w172]
                tunnel: [_ w170] -> w159
                tunnel: [w168 w169] -> w158
                tunnel: w161 -> [_ w169]
                tunnel: w160 -> [w168 _]
                frame False {
                }
                frame True {
                  n224 = String Subset(string=w172, offset (0)=1) -> (substring=w170:string)  [unwired: 1 in]
                }
              }
            }
            n225 = Array Size(array=w147) -> (size(s)=w148:i32)
            n226 = for {
              N: w148 -> [_]
              tunnel: w147 -> [w156] mode=indexing
              shift-right: [w155] -> w143
              shift-left: "" -> [w157]
              n227 = Concatenate Strings(w157, w156, "\r\n") -> (w155:string)
            }
            n228 = String Length(string=w143) -> (length=w142:i32)
            n229 = property on="Pending Tasks" class="LstBox (strict)"() -> ("Item Names"=w145:string[])  [unwired: 2 in, 2 out]
            n230 = Subtract(x=w142, y=4) -> (x-y=w141:i32)
            n231 = String Subset(string=w143, length (rest)=w141) -> (substring=w137:string)  [unwired: 1 in]
            n232 = property on="Tasks" class="Arr (strict)"() -> ("Value"=w151:string[][])  [unwired: 2 in, 2 out]
            n233 = Build Array (concatenate)(w137, w138) -> (w139:string[])
            n234 = Build Array (concatenate)(w145, w137) -> (w144:string[])
            n235 = Build Array (concatenate)(w151, w139) -> (w150:string[][])
            n236 = property on="Pending Tasks" class="LstBox (strict)"("Item Names"=w144) -> ()  [unwired: 2 in, 2 out]
            n237 = property on="Tasks" class="Arr (strict)"("Value"=w150) -> ()  [unwired: 2 in, 2 out]
          }
        }
      }
      n238 = while {
        stop <- w369 stop-if-true
        # "This loop handles the actual scanning algorithm."
        n239 = property on="QUIT" class="LVObjRef (strict)"() -> ("Value"=w368:refnum<vi>)  [unwired: 2 in, 2 out]
        n240 = property class="Bool (strict)"(reference=w368) -> ("Value"=w369:bool)  [unwired: 1 in, 2 out]
        n241 = property on="EMERGENCY" class="LVObjRef (strict)"() -> ("Value"=w364:refnum<vi>)  [unwired: 2 in, 2 out]
        n242 = property class="Bool (strict)"(reference=w364) -> ("Value"=w366:bool)  [unwired: 1 in, 2 out]
        n243 = property on="Scan in Progress" class="LVObjRef (strict)"() -> ("Value"=w365:refnum<vi>)  [unwired: 2 in, 2 out]
        n244 = property class="Bool (strict)"(reference=w365) -> ("Value"=w363:bool)  [unwired: 1 in, 2 out]
        n245 = Not(x=w366) -> (.not. x?=w362:bool)
        n246 = And(x=w363, y=w362) -> (x .and. y?=w367:bool)
        n247 = case shown="True" w367 {
          tunnel: w362 -> [w370 _]
          frame False {
            n248 = case shown="True" w370 {
              frame False {
              }
              frame True {
                n249 = property on="ABORT" class="Bool (strict)"("Value"=FALSE ("ABORT")) -> ()  [unwired: 2 in, 2 out]
              }
            }
          }
          frame True {
            # "Enter this structure if there's a scan running and no emergency."
            n250 = property on="Tasks" class="Arr (strict)"() -> ("Value"=w372:string[][])  [unwired: 2 in, 2 out]
            n251 = property on="Current Task" class="Arr (strict)"() -> ("Value"=w373:string[])  [unwired: 2 in, 2 out]
            n252 = Array Size(array=w372) -> (size(s)=w378:i32[])
            n253 = Array Size(array=w373) -> (size(s)=w376:i32)
            n254 = Index Array(array=w378, index=0) -> (element=w379:i32)
            n255 = Equal To 0?(x=w379) -> (x = 0?=w375:bool)
            n256 = Equal To 0?(x=w376) -> (x = 0?=w374:bool)
            n257 = And(x=w375, y=w374) -> (x .and. y?=w377:bool)
            n258 = case shown="False" w377 {
              tunnel: w374 -> [w382 _]
              tunnel: w373 -> [w381 _]
              frame False {
                # "Enter this structure if NOT (<Current Task> is empty AND <Tasks> is empty).  i.e. <Current Task> or <Tasks> has at least one element left to execute."
                n259 = flat-sequence {
                  tunnel: w382 -> [w402]
                  tunnel: w381 -> [w401]
                  frame #0 {
                    # "Pop the top element off <Current Task> and write it to <Current Action> for display to the user."
                    n260 = case shown="True" w402 {
                      tunnel: [w726 w730] -> w393
                      tunnel: w401 -> [w726 _]
                      frame False {
                      }
                      frame True {
                        w750 = "#" ("string")
                        w760 = "#" ("string")
                        w758 = "\r\n"
                        # "Order of execution:\n-Pop the top row off of <Tasks> and set it to <Current Task>.\n-Overwrite <Pending Tasks> with the first column of <Tasks>.\n-Pop the first element off of <Current Tasks> (should contain meta data) and display it to the user in <Current Scan>.\n-Use the \"File Name Gen\" subVI to calculate the output data file name.\n-Generate the header for the output file using the filename, the current time, and the meta data in <Current Scan>.\n-Open the file, write the header, then close the file.\n-Generate the first 2 columns of \"data\" (really, it's more header).  The first column is the long names of the independent variables and observables.  The second column is the short names.  Note that a \"#\" is added to the beginning of each column to indicate that it's a header.\n-Write the first 2 columns to the file using the \"Write to Spreadsheet File\" subVI.\n-Output <Current Task> from the structure, with blank entries removed."
                        # "Enter this structure if <Current Task> is empty."
                        # "Make new file"
                        # "Make file header"
                        n261 = property on="Tasks" class="Arr (strict)"() -> ("Value"=w736:string[][])  [unwired: 2 in, 2 out]
                        n262 = Delete From Array(array=w736, index (row)=0) -> (deleted portion=w770:string[], array with subset deleted=w772:string[][])  [unwired: 2 in]
                        n263 = property on="Tasks" class="Arr (strict)"("Value"=w772) -> ()  [unwired: 2 in, 2 out]
                        n264 = property on="Current Task" class="Arr (strict)"("Value"=w770) -> ()  [unwired: 2 in, 2 out]
                        n265 = Concatenate Strings(w758, w760) -> (w757:string)
                        n266 = Delete From Array(array=w772, index (col)=0 ("disabled index (col)")) -> (deleted portion=w771:string[])  [unwired: 2 in, 1 out]
                        n267 = Delete From Array(array=w770, index=0) -> (deleted portion=w761:string, array with subset deleted=w735:string[])  [unwired: 1 in]
                        "Current Scan" <- w761
                        n268 = property on="Pending Tasks" class="LstBox (strict)"("Item Names"=w771) -> ()  [unwired: 2 in, 2 out]
                        n269 = Search and Replace String(replace all?=TRUE ("replace all? (F)"), input string=w761, search string=w758, replace string=w757) -> (result string=w756:string)  [unwired: 4 in, 3 out]
                        n270 = call "filename generator (number).vi"("create folder?"=TRUE, "digits (2)"="Number of Digits in Output Filename Suffix", "separator (none)"="Spacer in Output Filenames", "start number (0)"="Start Counting From...", "extension"="Output File Extension", "filename root"="Output Filename", "root folder"="Folder") -> ("filename"=w773:path)  [unwired: 3 in, 1 out]
                        "Current File" <- w773
                        n271 = Array Size(array=w735) -> (size(s)=w734:i32)
                        n272 = Strip Path(path=w773) -> (name=w783:string)  [unwired: 1 out]
                        n273 = Initialize Array("" ("element"), 0 ("dimension size")) -> (w731:string[])
                        n274 = Get Date/Time String(want seconds? (F)=TRUE) -> (date string=w781:string, time string=w779:string)  [unwired: 2 in]
                        n275 = for {
                          N: w734 -> [_]
                          tunnel: w735 -> [w802]
                          shift-right: [w797] -> w730
                          shift-left: w731 -> [w801]
                          i -> [w803]
                          n276 = Index Array(array=w802, index=w803) -> (element=w796:string)
                          n277 = property on="Character That Separates Parameters in Scan Commands" class="Str"() -> ("Value"=w804:string)  [unwired: 2 in, 2 out]
                          n278 = Search/Split String(string=w796, search string/char (-)=w804) -> (substring before match=w800:string)  [unwired: 1 in, 2 out]
                          n279 = Equal?(x="" ("element"), y=w800) -> (x = y?=w798:bool)
                          n280 = case shown="False" w798 {
                            tunnel: w801 -> [w807 w808]
                            tunnel: [w806 w808] -> w797
                            tunnel: w796 -> [w805 _]
                            frame False {
                              n281 = Build Array (concatenate)(w807, w805) -> (w806:string[])
                            }
                            frame True {
                            }
                          }
                        }
                        n282 = call <vilib>:"Space Constant.vi"() -> ("String"=w780:string)
                        n283 = property on="Error" class="LVObjRef (strict)"() -> ("Value"=w764:refnum<vi>)  [unwired: 2 in, 2 out]
                        n284 = Concatenate Strings(w760, w783, w758, w760, w781, w780, w779, w758, w760, w756, w758) -> (w778:string)
                        n285 = property class="Clust (strict)"(reference=w764) -> (reference out=w765:refnum<vi>, "Value"=w767:errorcluster)  [unwired: 1 in, 1 out]
                        n286 = property on="Independent Variables" class="Arr (strict)"() -> ("Value"=w752:string[][])  [unwired: 2 in, 2 out]
                        n287 = property on="Observables" class="Arr (strict)"() -> ("Value"=w745:string[][])  [unwired: 2 in, 2 out]
                        n288 = Open/Create/Replace File(file path (use dialog)=w773, error in=w767, operation (0:open)=T2."create") -> (refnum out=w789:refnum<file>, error out=w788:errorcluster)  [unwired: 3 in, 1 out]
                        n289 = Write to Text File(file (use dialog)=w789, text=w778, error in=w788) -> (refnum out=w787:refnum<file>, error out=w786:errorcluster)  [unwired: 1 in, 1 out]
                        n290 = Delete From Array(array=w752, index (row)=0) -> (deleted portion=w737:string[])  [unwired: 2 in, 1 out]
                        n291 = Index Array(array=w745, index (row)=0) -> (element=w762:string[])  [unwired: 1 in]
                        n292 = Delete From Array(array=w752, index (row)=1) -> (deleted portion=w738:string[])  [unwired: 2 in, 1 out]
                        n293 = Index Array(array=w745, index (row)=1) -> (element=w743:string[])  [unwired: 1 in]
                        n294 = Close File(refnum=w787, error in=w786) -> (path=w795:path, error out=w766:errorcluster)
                        n295 = property class="Clust (strict)"(reference=w765, "Value"=w766) -> ()  [unwired: 1 in, 2 out]
                        n296 = Concatenate Strings(w750, "time") -> (w749:string)
                        n297 = Concatenate Strings(w750, "Timestamp (sec)") -> (w755:string)
                        n298 = Array Size(array=w730) -> (size(s)=w729:i32)
                        n299 = Insert Into Array(array=w737, index=0, new element=w755) -> (w753:string[])
                        n300 = Insert Into Array(array=w753, new element=w762) -> (w747:string[])  [unwired: 1 in]
                        n301 = Insert Into Array(array=w738, index=0, new element=w749) -> (w742:string[])
                        n302 = Subtract(x=w729, y=1) -> (x-y=→"Total Actions":i32)
                        n303 = Insert Into Array(array=w742, new element=w743) -> (w741:string[])  [unwired: 1 in]
                        n304 = Build Array(w747, w741) -> (w746:string[][])
                        n305 = call-poly <vilib>:"Write To Spreadsheet File.vi"("append to file? (new file:F)"=TRUE, "2D data"=w746, "file path (dialog if empty)"=w795) -> ()  [unwired: 5 in, 1 out]
                      }
                    }
                    n306 = property on="Status" class="Str"("Value"="Scanning" ("Status")) -> ()  [unwired: 2 in, 2 out]
                    n307 = Array Size(array=w393) -> (size(s)=w392:i32)
                    n308 = property on="Total Actions" class="DigNum (strict)"() -> ("Value"=w391:i32)  [unwired: 2 in, 2 out]
                    n309 = Divide(x=w392, y=w391) -> (x/y=w389:dbl)
                    n310 = Subtract(x=1, y=w389) -> (x-y=w387:dbl)
                    n311 = Multiply(x=w387, y=100) -> (x*y=w386:dbl)
                    n312 = To Long Integer(number=w386) -> (32bit integer=w384:i32)
                    n313 = Greater Than 0?(x=w384) -> (x > 0?=w385:bool)
                    n314 = case shown="False" w385 {
                      tunnel: w384 -> [_ w404]
                      tunnel: [0 w404] -> w383
                      frame False {
                      }
                      frame True {
                      }
                    }
                    "Progress:" <- w383
                    n315 = Delete From Array(array=w393, index=0) -> (deleted portion=w399:string, array with subset deleted=w396:string[])  [unwired: 1 in]
                    "Current Action" <- w399
                    n316 = property on="Current Task" class="Arr (strict)"("Value"=w396) -> ()  [unwired: 2 in, 2 out]
                    n317 = Search/Split String(string=w399, search string/char (-)="Character That Separates Parameters in Scan Commands") -> (substring before match=w395:string, match + rest of string=w398:string)  [unwired: 1 in, 1 out]
                    n318 = case shown="\"measure\"" w395 {
                      tunnel: w398 -> [w406 w545 _ w722 _]
                      tunnel: "Character That Separates Parameters in Scan Commands" -> [w405 w546 _ _ _]
                      frame "set" {
                        n319 = flat-sequence {
                          tunnel: w406 -> [w408]
                          tunnel: w405 -> [w407]
                          frame #0 {
                            n320 = while {
                              shift-right: [w413] -> _
                              shift-left: w408 -> [w419]
                              tunnel: w407 -> [w411]
                              stop <- w414 stop-if-true
                              n321 = String Subset(string=w419, offset (0)=1) -> (substring=w421:string)  [unwired: 1 in]
                              n322 = property on="Current Task" class="Arr (strict)"() -> ("Value"=w410:string[])  [unwired: 2 in, 2 out]
                              n323 = Search/Split String(string=w421, search string/char (-)=w411) -> (substring before match=w422:string, match + rest of string=w423:string)  [unwired: 1 in, 1 out]
                              n324 = String Subset(string=w423, offset (0)=1) -> (substring=w412:string)  [unwired: 1 in]
                              n325 = Delete From Array(array=w410, index=0) -> (deleted portion=w417:string, array with subset deleted=w409:string[])  [unwired: 1 in]
                              n326 = case shown="\"vb\"" w422 {
                                tunnel: w412 -> [_ w426 w431 w436 w441 w446 w450 w454 w458 w462 w466 w470 w474 w478 w482 w486 w489 w492 w495 w498 w501 w504 w507 w510 w513 w515 w519]
                                frame "error", Default {
                                }
                                frame "dummy" {
                                n327 = Fract/Exp String To Number(string=w426) -> (number=w425:dbl)  [unwired: 3 in, 1 out]
                                n328 = property on="Dummy" class="DigNum (strict)"("Value"=w425) -> ()  [unwired: 2 in, 2 out]
                                }
                                frame "xpos" {
                                w429 = TRUE ("Measuring")
                                n329 = property on="X Go" class="LVObjRef (strict)"() -> ("Value"=w428:refnum<vi>)  [unwired: 2 in, 2 out]
                                n330 = Fract/Exp String To Number(string=w431) -> (number=w430:dbl)  [unwired: 3 in, 1 out]
                                n331 = property class="Bool (strict)"(reference=w428, "Value"=w429) -> ()  [unwired: 1 in, 2 out]
                                n332 = property on="X Go To (mm)" class="LVObjRef (strict)"() -> ("Value"=w427:refnum<vi>)  [unwired: 2 in, 2 out]
                                n333 = property class="DigNum (strict)"(reference=w427, "Value"=w430) -> ()  [unwired: 1 in, 2 out]
                                "Set Motors?" <- w429
                                }
                                frame "ypos" {
                                w434 = TRUE ("Y Go?")
                                n334 = property on="Y Go" class="LVObjRef (strict)"() -> ("Value"=w433:refnum<vi>)  [unwired: 2 in, 2 out]
                                n335 = Fract/Exp String To Number(string=w436) -> (number=w435:dbl)  [unwired: 3 in, 1 out]
                                n336 = property on="Set Motors?" class="Bool (strict)"("Value"=w434) -> ()  [unwired: 2 in, 2 out]
                                n337 = property class="Bool (strict)"(reference=w433, "Value"=w434) -> ()  [unwired: 1 in, 2 out]
                                n338 = property on="Y Go To (mm)" class="LVObjRef (strict)"() -> ("Value"=w432:refnum<vi>)  [unwired: 2 in, 2 out]
                                n339 = property class="DigNum (strict)"(reference=w432, "Value"=w435) -> ()  [unwired: 1 in, 2 out]
                                }
                                frame "zpos" {
                                w439 = TRUE ("Z Go?")
                                n340 = property on="Z Go" class="LVObjRef (strict)"() -> ("Value"=w438:refnum<vi>)  [unwired: 2 in, 2 out]
                                n341 = Fract/Exp String To Number(string=w441) -> (number=w440:dbl)  [unwired: 3 in, 1 out]
                                n342 = property on="Set Motors?" class="Bool (strict)"("Value"=w439) -> ()  [unwired: 2 in, 2 out]
                                n343 = property class="Bool (strict)"(reference=w438, "Value"=w439) -> ()  [unwired: 1 in, 2 out]
                                n344 = property on="Z Go To (mm)" class="LVObjRef (strict)"() -> ("Value"=w437:refnum<vi>)  [unwired: 2 in, 2 out]
                                n345 = property class="DigNum (strict)"(reference=w437, "Value"=w440) -> ()  [unwired: 1 in, 2 out]
                                }
                                frame "theta" {
                                w444 = TRUE ("Theta Go?")
                                n346 = Fract/Exp String To Number(string=w446) -> (number=w445:dbl)  [unwired: 3 in, 1 out]
                                n347 = property on="Theta Go" class="LVObjRef (strict)"() -> ("Value"=w443:refnum<vi>)  [unwired: 2 in, 2 out]
                                n348 = property class="Bool (strict)"(reference=w443, "Value"=w444) -> ()  [unwired: 1 in, 2 out]
                                n349 = property on="Set Motors?" class="Bool (strict)"("Value"=w444) -> ()  [unwired: 2 in, 2 out]
                                n350 = property on="Theta Go To (mm)" class="LVObjRef (strict)"() -> ("Value"=w442:refnum<vi>)  [unwired: 2 in, 2 out]
                                n351 = property class="DigNum (strict)"(reference=w442, "Value"=w445) -> ()  [unwired: 1 in, 2 out]
                                }
                                frame "grid" {
                                n352 = Fract/Exp String To Number(string=w450) -> (number=w449:dbl)  [unwired: 3 in, 1 out]
                                n353 = property on="EG Grid (V)" class="LVObjRef (strict)"() -> ("Value"=w447:refnum<vi>)  [unwired: 2 in, 2 out]
                                n354 = property class="DigNum (strict)"(reference=w447, "Value"=w449) -> ()  [unwired: 1 in, 2 out]
                                "Set EG?" <- TRUE ("Set EG?")
                                }
                                frame "en" {
                                n355 = Fract/Exp String To Number(string=w454) -> (number=w453:dbl)  [unwired: 3 in, 1 out]
                                n356 = property on="Set EG?" class="Bool (strict)"("Value"=TRUE) -> ()  [unwired: 2 in, 2 out]
                                n357 = property on="EG Energy (eV)" class="LVObjRef (strict)"() -> ("Value"=w451:refnum<vi>)  [unwired: 2 in, 2 out]
                                n358 = property class="DigNum (strict)"(reference=w451, "Value"=w453) -> ()  [unwired: 1 in, 2 out]
                                }
                                frame "ext" {
                                n359 = Fract/Exp String To Number(string=w458) -> (number=w457:dbl)  [unwired: 3 in, 1 out]
                                n360 = property on="Set EG?" class="Bool (strict)"("Value"=TRUE) -> ()  [unwired: 2 in, 2 out]
                                n361 = property on="EG Extraction (V)" class="LVObjRef (strict)"() -> ("Value"=w455:refnum<vi>)  [unwired: 2 in, 2 out]
                                n362 = property class="DigNum (strict)"(reference=w455, "Value"=w457) -> ()  [unwired: 1 in, 2 out]
                                }
                                frame "f1" {
                                n363 = Fract/Exp String To Number(string=w462) -> (number=w461:dbl)  [unwired: 3 in, 1 out]
                                n364 = property on="Set EG?" class="Bool (strict)"("Value"=TRUE) -> ()  [unwired: 2 in, 2 out]
                                n365 = property on="EG Focus 1 (V)" class="LVObjRef (strict)"() -> ("Value"=w459:refnum<vi>)  [unwired: 2 in, 2 out]
                                n366 = property class="DigNum (strict)"(reference=w459, "Value"=w461) -> ()  [unwired: 1 in, 2 out]
                                }
                                frame "f2" {
                                n367 = Fract/Exp String To Number(string=w466) -> (number=w465:dbl)  [unwired: 3 in, 1 out]
                                n368 = property on="Set EG?" class="Bool (strict)"("Value"=TRUE) -> ()  [unwired: 2 in, 2 out]
                                n369 = property on="EG Focus 2 (V)" class="LVObjRef (strict)"() -> ("Value"=w463:refnum<vi>)  [unwired: 2 in, 2 out]
                                n370 = property class="DigNum (strict)"(reference=w463, "Value"=w465) -> ()  [unwired: 1 in, 2 out]
                                }
                                frame "fil" {
                                n371 = Fract/Exp String To Number(string=w470) -> (number=w469:dbl)  [unwired: 3 in, 1 out]
                                n372 = property on="Set EG?" class="Bool (strict)"("Value"=TRUE) -> ()  [unwired: 2 in, 2 out]
                                n373 = property on="EG Filament (V)" class="LVObjRef (strict)"() -> ("Value"=w467:refnum<vi>)  [unwired: 2 in, 2 out]
                                n374 = property class="DigNum (strict)"(reference=w467, "Value"=w469) -> ()  [unwired: 1 in, 2 out]
                                }
                                frame "x1" {
                                n375 = Fract/Exp String To Number(string=w474) -> (number=w473:dbl)  [unwired: 3 in, 1 out]
                                n376 = property on="Set EG?" class="Bool (strict)"("Value"=TRUE) -> ()  [unwired: 2 in, 2 out]
                                n377 = property on="EG X1 Alignment (V)" class="LVObjRef (strict)"() -> ("Value"=w471:refnum<vi>)  [unwired: 2 in, 2 out]
                                n378 = property class="DigNum (strict)"(reference=w471, "Value"=w473) -> ()  [unwired: 1 in, 2 out]
                                }
                                frame "x2" {
                                n379 = Fract/Exp String To Number(string=w478) -> (number=w477:dbl)  [unwired: 3 in, 1 out]
                                n380 = property on="Set EG?" class="Bool (strict)"("Value"=TRUE) -> ()  [unwired: 2 in, 2 out]
                                n381 = property on="EG X2 Alignment (V)" class="LVObjRef (strict)"() -> ("Value"=w475:refnum<vi>)  [unwired: 2 in, 2 out]
                                n382 = property class="DigNum (strict)"(reference=w475, "Value"=w477) -> ()  [unwired: 1 in, 2 out]
                                }
                                frame "y1" {
                                n383 = Fract/Exp String To Number(string=w482) -> (number=w481:dbl)  [unwired: 3 in, 1 out]
                                n384 = property on="Set EG?" class="Bool (strict)"("Value"=TRUE) -> ()  [unwired: 2 in, 2 out]
                                n385 = property on="EG Y1 Alignment (V)" class="LVObjRef (strict)"() -> ("Value"=w479:refnum<vi>)  [unwired: 2 in, 2 out]
                                n386 = property class="DigNum (strict)"(reference=w479, "Value"=w481) -> ()  [unwired: 1 in, 2 out]
                                }
                                frame "y2" {
                                n387 = Fract/Exp String To Number(string=w486) -> (number=w485:dbl)  [unwired: 3 in, 1 out]
                                n388 = property on="Set EG?" class="Bool (strict)"("Value"=TRUE) -> ()  [unwired: 2 in, 2 out]
                                n389 = property on="EG Y2 Alignment (V)" class="LVObjRef (strict)"() -> ("Value"=w483:refnum<vi>)  [unwired: 2 in, 2 out]
                                n390 = property class="DigNum (strict)"(reference=w483, "Value"=w485) -> ()  [unwired: 1 in, 2 out]
                                }
                                frame "6485s" {
                                n391 = Fract/Exp String To Number(string=w489) -> (number=w487:dbl)  [unwired: 3 in, 1 out]
                                n392 = property on="6485 Samples/measurement" class="LVObjRef (strict)"() -> ("Value"=w488:refnum<vi>)  [unwired: 2 in, 2 out]
                                n393 = property class="DigNum (strict)"(reference=w488, "Value"=w487) -> ()  [unwired: 1 in, 2 out]
                                }
                                frame "6487s" {
                                n394 = Fract/Exp String To Number(string=w492) -> (number=w490:dbl)  [unwired: 3 in, 1 out]
                                n395 = property on="6487 Samples/measurement" class="LVObjRef (strict)"() -> ("Value"=w491:refnum<vi>)  [unwired: 2 in, 2 out]
                                n396 = property class="DigNum (strict)"(reference=w491, "Value"=w490) -> ()  [unwired: 1 in, 2 out]
                                }
                                frame "6487v" {
                                n397 = Fract/Exp String To Number(string=w495) -> (number=w494:dbl)  [unwired: 3 in, 1 out]
                                n398 = property on="Keithley6487 Potential (V)" class="LVObjRef (strict)"() -> ("Value"=w493:refnum<vi>)  [unwired: 2 in, 2 out]
                                n399 = property class="DigNum (strict)"(reference=w493, "Value"=w494) -> ()  [unwired: 1 in, 2 out]
                                }
                                frame "gm2dw" {
                                n400 = Fract/Exp String To Number(string=w498) -> (number=w497:dbl)  [unwired: 3 in, 1 out]
                                n401 = property on="GM2 Dwell" class="LVObjRef (strict)"() -> ("Value"=w496:refnum<vi>)  [unwired: 2 in, 2 out]
                                n402 = property class="DigNum (strict)"(reference=w496, "Value"=w497) -> ()  [unwired: 1 in, 2 out]
                                }
                                frame "gm2ll" {
                                n403 = Fract/Exp String To Number(string=w501) -> (number=w500:dbl)  [unwired: 3 in, 1 out]
                                n404 = property on="GM2 LLD" class="LVObjRef (strict)"() -> ("Value"=w499:refnum<vi>)  [unwired: 2 in, 2 out]
                                n405 = property class="DigNum (strict)"(reference=w499, "Value"=w500) -> ()  [unwired: 1 in, 2 out]
                                }
                                frame "gm2ul" {
                                n406 = Fract/Exp String To Number(string=w504) -> (number=w503:dbl)  [unwired: 3 in, 1 out]
                                n407 = property on="GM2 ULD" class="LVObjRef (strict)"() -> ("Value"=w502:refnum<vi>)  [unwired: 2 in, 2 out]
                                n408 = property class="DigNum (strict)"(reference=w502, "Value"=w503) -> ()  [unwired: 1 in, 2 out]
                                }
                                frame "gm1dw" {
                                n409 = Fract/Exp String To Number(string=w507) -> (number=w506:dbl)  [unwired: 3 in, 1 out]
                                n410 = property on="GM1 Dwell" class="LVObjRef (strict)"() -> ("Value"=w505:refnum<vi>)  [unwired: 2 in, 2 out]
                                n411 = property class="DigNum (strict)"(reference=w505, "Value"=w506) -> ()  [unwired: 1 in, 2 out]
                                }
                                frame "gm1ll" {
                                n412 = Fract/Exp String To Number(string=w510) -> (number=w509:dbl)  [unwired: 3 in, 1 out]
                                n413 = property on="GM1 LLD" class="LVObjRef (strict)"() -> ("Value"=w508:refnum<vi>)  [unwired: 2 in, 2 out]
                                n414 = property class="DigNum (strict)"(reference=w508, "Value"=w509) -> ()  [unwired: 1 in, 2 out]
                                }
                                frame "gm1ul" {
                                n415 = Fract/Exp String To Number(string=w513) -> (number=w512:dbl)  [unwired: 3 in, 1 out]
                                n416 = property on="GM1 ULD" class="LVObjRef (strict)"() -> ("Value"=w511:refnum<vi>)  [unwired: 2 in, 2 out]
                                n417 = property class="DigNum (strict)"(reference=w511, "Value"=w512) -> ()  [unwired: 1 in, 2 out]
                                }
                                frame "va" {
                                n418 = Fract/Exp String To Number(string=w515) -> (number=w514:dbl)  [unwired: 3 in, 1 out]
                                n419 = property on="Voltage Supply A" class="LVObjRef (strict)"() -> ("Value"=w516:refnum<vi>)  [unwired: 2 in, 2 out]
                                n420 = property class="DigNum (strict)"(reference=w516, "Value"=w514) -> ()  [unwired: 1 in, 2 out]
                                "Set VA?" <- TRUE ("Set VA?")
                                }
                                frame "vb" {
                                n421 = Fract/Exp String To Number(string=w519) -> (number=w518:dbl)  [unwired: 3 in, 1 out]
                                n422 = property on="Voltage Supply B" class="LVObjRef (strict)"() -> ("Value"=w520:refnum<vi>)  [unwired: 2 in, 2 out]
                                n423 = property class="DigNum (strict)"(reference=w520, "Value"=w518) -> ()  [unwired: 1 in, 2 out]
                                "Set VB?" <- TRUE ("Set VB?")
                                }
                              }
                              n424 = Search/Split String(string=w417, search string/char (-)=w411) -> (substring before match=w416:string, match + rest of string=w413:string)  [unwired: 1 in, 1 out]
                              n425 = property on="Current Task" class="Arr (strict)"("Value"=w409) -> ()  [unwired: 2 in, 2 out]
                              n426 = property on="Current Action" class="Str"("Value"=w417) -> ()  [unwired: 2 in, 2 out]
                              n427 = Not Equal?(x=w416, y="set") -> (x != y?=w414:bool)
                            }
                          }
                          frame #1 {
                            n428 = property on="Set EG?" class="Bool (strict)"() -> ("Value"=w524:bool)  [unwired: 2 in, 2 out]
                            n429 = property on="Set VB?" class="Bool (strict)"() -> ("Value"=w522:bool)  [unwired: 2 in, 2 out]
                            n430 = property on="Set VA?" class="Bool (strict)"() -> ("Value"=w523:bool)  [unwired: 2 in, 2 out]
                            n431 = property on="Set Motors?" class="Bool (strict)"() -> ("Value"=w525:bool)  [unwired: 2 in, 2 out]
                            n432 = case shown="True" w524 {
                              frame False {
                              }
                              frame True {
                                n433 = property on="Set EG" class="LVObjRef (strict)"() -> ("Value"=w530:refnum<vi>)  [unwired: 2 in, 2 out]
                                n434 = property class="Bool (strict)"(reference=w530, "Value"=TRUE) -> ()  [unwired: 1 in, 2 out]
                              }
                            }
                            n435 = case shown="True" w522 {
                              frame False {
                              }
                              frame True {
                                n436 = property on="Set VB" class="LVObjRef (strict)"() -> ("Value"=w527:refnum<vi>)  [unwired: 2 in, 2 out]
                                n437 = property class="Bool (strict)"(reference=w527, "Value"=TRUE) -> ()  [unwired: 1 in, 2 out]
                              }
                            }
                            n438 = case shown="True" w523 {
                              frame False {
                              }
                              frame True {
                                n439 = property on="Set VA" class="LVObjRef (strict)"() -> ("Value"=w529:refnum<vi>)  [unwired: 2 in, 2 out]
                                n440 = property class="Bool (strict)"(reference=w529, "Value"=TRUE) -> ()  [unwired: 1 in, 2 out]
                              }
                            }
                            n441 = case shown="True" w525 {
                              frame False {
                              }
                              frame True {
                                n442 = property on="Set Motors" class="LVObjRef (strict)"() -> ("Value"=w532:refnum<vi>)  [unwired: 2 in, 2 out]
                                n443 = property class="Bool (strict)"(reference=w532, "Value"=TRUE) -> ()  [unwired: 1 in, 2 out]
                              }
                            }
                          }
                          frame #2 {
                            n444 = while {
                              stop <- w542 stop-if-true
                              n445 = property on="Set VA" class="LVObjRef (strict)"() -> ("Value"=w540:refnum<vi>)  [unwired: 2 in, 2 out]
                              n446 = property on="Set VB" class="LVObjRef (strict)"() -> ("Value"=w539:refnum<vi>)  [unwired: 2 in, 2 out]
                              n447 = property on="ABORT" class="Bool (strict)"() -> ("Value"=w541:bool)  [unwired: 2 in, 2 out]
                              n448 = property on="Set Motors" class="LVObjRef (strict)"() -> ("Value"=w544:refnum<vi>)  [unwired: 2 in, 2 out]
                              n449 = property on="Set EG" class="LVObjRef (strict)"() -> ("Value"=w543:refnum<vi>)  [unwired: 2 in, 2 out]
                              n450 = property class="Bool (strict)"(reference=w539) -> ("Value"=w535:bool)  [unwired: 1 in, 2 out]
                              n451 = property class="Bool (strict)"(reference=w540) -> ("Value"=w536:bool)  [unwired: 1 in, 2 out]
                              n452 = property class="Bool (strict)"(reference=w544) -> ("Value"=w538:bool)  [unwired: 1 in, 2 out]
                              n453 = property class="Bool (strict)"(reference=w543) -> ("Value"=w537:bool)  [unwired: 1 in, 2 out]
                              n454 = Compound Arithmetic op=OR(w538, w537, w536, w535) -> (invert w534:bool)
                              n455 = Or(x=w534, y=w541) -> (x .or. y?=w542:bool)
                            }
                          }
                        }
                      }
                      frame "measure" {
                        n456 = flat-sequence {
                          tunnel: w546 -> [w564]
                          tunnel: w545 -> [w563]
                          frame #0 {
                            n457 = while {
                              stop <- w562 continue-if-true
                              # "Wait for the motors to stop moving."
                              n458 = property on="Motors Are Active" class="LVObjRef (strict)"() -> ("Value"=w561:refnum<vi>)  [unwired: 2 in, 2 out]
                              n459 = property class="Bool (strict)"(reference=w561) -> ("Value"=w562:bool)  [unwired: 1 in, 2 out]
                            }
                            n460 = while {
                              stop <- w555 stop-if-true
                              # "Waiting for measurements to finish."
                              n461 = property on="Measure 6485" class="LVObjRef (strict)"() -> ("Value"=w560:refnum<vi>)  [unwired: 2 in, 2 out]
                              n462 = property on="Measure 6487" class="LVObjRef (strict)"() -> ("Value"=w559:refnum<vi>)  [unwired: 2 in, 2 out]
                              n463 = property on="Measure GM1" class="LVObjRef (strict)"() -> ("Value"=w553:refnum<vi>)  [unwired: 2 in, 2 out]
                              n464 = property on="Measure GM2" class="LVObjRef (strict)"() -> ("Value"=w554:refnum<vi>)  [unwired: 2 in, 2 out]
                              n465 = property class="Bool (strict)"(reference=w560) -> ("Value"=w558:bool)  [unwired: 1 in, 2 out]
                              n466 = property class="Bool (strict)"(reference=w559) -> ("Value"=w557:bool)  [unwired: 1 in, 2 out]
                              n467 = property class="Bool (strict)"(reference=w553) -> ("Value"=w552:bool)  [unwired: 1 in, 2 out]
                              n468 = property class="Bool (strict)"(reference=w554) -> ("Value"=w551:bool)  [unwired: 1 in, 2 out]
                              n469 = Compound Arithmetic op=OR(w558, w557, w552, w551) -> (w550:bool)
                              n470 = property on="ABORT" class="Bool (strict)"() -> ("Value"=w556:bool)  [unwired: 2 in, 2 out]
                              n471 = Not(x=w550) -> (.not. x?=w549:bool)
                              n472 = Or(x=w549, y=w556) -> (x .or. y?=w555:bool)
                            }
                            n473 = Wait (ms)(milliseconds to wait="Settling time (ms)") -> ()  [unwired: 1 out]
                            "Status" <- "Waiting for Motors to Finish" ("Status")
                          }
                          frame #1 {
                            n474 = while {
                              shift-right: [w570] -> _
                              shift-left: w563 -> [w577]
                              tunnel: w564 -> [w567]
                              stop <- w571 stop-if-true
                              n475 = String Subset(string=w577, offset (0)=1) -> (substring=w566:string)  [unwired: 1 in]
                              n476 = Search/Split String(string=w566, search string/char (-)=w567) -> (substring before match=w565:string)  [unwired: 1 in, 2 out]
                              n477 = property on="Current Task" class="Arr (strict)"() -> ("Value"=w569:string[])  [unwired: 2 in, 2 out]
                              n478 = case shown="\"gm2\"" w565 {
                                frame "gm2" {
                                n479 = property on="Measure GM2" class="LVObjRef (strict)"() -> ("Value"=w579:refnum<vi>)  [unwired: 2 in, 2 out]
                                n480 = property class="Bool (strict)"(reference=w579, "Value"=TRUE) -> ()  [unwired: 1 in, 2 out]
                                }
                                frame "gm1" {
                                n481 = property on="Measure GM1" class="LVObjRef (strict)"() -> ("Value"=w581:refnum<vi>)  [unwired: 2 in, 2 out]
                                n482 = property class="Bool (strict)"(reference=w581, "Value"=TRUE) -> ()  [unwired: 1 in, 2 out]
                                }
                                frame "6485c" {
                                n483 = property on="Measure 6485" class="LVObjRef (strict)"() -> ("Value"=w582:refnum<vi>)  [unwired: 2 in, 2 out]
                                n484 = property class="Bool (strict)"(reference=w582, "Value"=TRUE ("Measure 6485")) -> ()  [unwired: 1 in, 2 out]
                                }
                                frame "6487c" {
                                n485 = property on="Measure 6487" class="LVObjRef (strict)"() -> ("Value"=w584:refnum<vi>)  [unwired: 2 in, 2 out]
                                n486 = property class="Bool (strict)"(reference=w584, "Value"=TRUE ("Measure 6485")) -> ()  [unwired: 1 in, 2 out]
                                }
                                frame "error", Default {
                                }
                              }
                              n487 = Delete From Array(array=w569, index=0) -> (deleted portion=w573:string, array with subset deleted=w568:string[])  [unwired: 1 in]
                              n488 = property on="Current Task" class="Arr (strict)"("Value"=w568) -> ()  [unwired: 2 in, 2 out]
                              n489 = property on="Current Action" class="Str"("Value"=w573) -> ()  [unwired: 2 in, 2 out]
                              n490 = Search/Split String(string=w573, search string/char (-)=w567) -> (substring before match=w574:string, match + rest of string=w570:string)  [unwired: 1 in, 1 out]
                              n491 = Not Equal?(x=w574, y="measure") -> (x != y?=w571:bool)
                            }
                          }
                          frame #2 {
                            n492 = while {
                              stop <- w592 stop-if-true
                              # "Waiting for measurements to finish."
                              n493 = property on="Measure 6485" class="LVObjRef (strict)"() -> ("Value"=w597:refnum<vi>)  [unwired: 2 in, 2 out]
                              n494 = property on="Measure 6487" class="LVObjRef (strict)"() -> ("Value"=w596:refnum<vi>)  [unwired: 2 in, 2 out]
                              n495 = property on="Measure GM1" class="LVObjRef (strict)"() -> ("Value"=w590:refnum<vi>)  [unwired: 2 in, 2 out]
                              n496 = property on="Measure GM2" class="LVObjRef (strict)"() -> ("Value"=w591:refnum<vi>)  [unwired: 2 in, 2 out]
                              n497 = property class="Bool (strict)"(reference=w597) -> ("Value"=w595:bool)  [unwired: 1 in, 2 out]
                              n498 = property class="Bool (strict)"(reference=w596) -> ("Value"=w594:bool)  [unwired: 1 in, 2 out]
                              n499 = property class="Bool (strict)"(reference=w590) -> ("Value"=w589:bool)  [unwired: 1 in, 2 out]
                              n500 = property class="Bool (strict)"(reference=w591) -> ("Value"=w588:bool)  [unwired: 1 in, 2 out]
                              n501 = Compound Arithmetic op=OR(w595, w594, w589, w588) -> (w587:bool)
                              n502 = property on="ABORT" class="Bool (strict)"() -> ("Value"=w593:bool)  [unwired: 2 in, 2 out]
                              n503 = Not(x=w587) -> (.not. x?=w586:bool)
                              n504 = Or(x=w586, y=w593) -> (x .or. y?=w592:bool)
                            }
                          }
                          frame #3 {
                            # "Update the output file."
                            n505 = Get Date/Time In Seconds() -> (seconds since 1Jan1904=w607:timestamp)
                            n506 = To Double Precision Float(number=w607) -> (double precision float=w606:dbl)
                            n507 = Number To Fractional String(number=w606) -> (F-format string=w605:string)  [unwired: 3 in]
                            n508 = Number To Fractional String(number="Dummy") -> (F-format string=w598:string)  [unwired: 3 in]
                            n509 = property on="X (mm)" class="LVObjRef (strict)"() -> ("Value"=w643:refnum<vi>)  [unwired: 2 in, 2 out]
                            n510 = property on="Y (mm)" class="LVObjRef (strict)"() -> ("Value"=w642:refnum<vi>)  [unwired: 2 in, 2 out]
                            n511 = property on="Z (mm)" class="LVObjRef (strict)"() -> ("Value"=w640:refnum<vi>)  [unwired: 2 in, 2 out]
                            n512 = property on="Keithley6487 Potential (V)" class="LVObjRef (strict)"() -> ("Value"=w646:refnum<vi>)  [unwired: 2 in, 2 out]
                            n513 = property on="Theta (deg)" class="LVObjRef (strict)"() -> ("Value"=w639:refnum<vi>)  [unwired: 2 in, 2 out]
                            n514 = property on="EG Grid (V)" class="LVObjRef (strict)"() -> ("Value"=w671:refnum<vi>)  [unwired: 2 in, 2 out]
                            n515 = property on="EG Energy (eV)" class="LVObjRef (strict)"() -> ("Value"=w673:refnum<vi>)  [unwired: 2 in, 2 out]
                            n516 = property on="EG Extraction (V)" class="LVObjRef (strict)"() -> ("Value"=w675:refnum<vi>)  [unwired: 2 in, 2 out]
                            n517 = property on="EG Focus 1 (V)" class="LVObjRef (strict)"() -> ("Value"=w677:refnum<vi>)  [unwired: 2 in, 2 out]
                            n518 = property on="EG Focus 2 (V)" class="LVObjRef (strict)"() -> ("Value"=w679:refnum<vi>)  [unwired: 2 in, 2 out]
                            n519 = property on="EG Filament (V)" class="LVObjRef (strict)"() -> ("Value"=w682:refnum<vi>)  [unwired: 2 in, 2 out]
                            n520 = property on="EG X1 Alignment (V)" class="LVObjRef (strict)"() -> ("Value"=w683:refnum<vi>)  [unwired: 2 in, 2 out]
                            n521 = property on="EG X2 Alignment (V)" class="LVObjRef (strict)"() -> ("Value"=w685:refnum<vi>)  [unwired: 2 in, 2 out]
                            n522 = property on="EG Y1 Alignment (V)" class="LVObjRef (strict)"() -> ("Value"=w687:refnum<vi>)  [unwired: 2 in, 2 out]
                            n523 = property on="EG Y2 Alignment (V)" class="LVObjRef (strict)"() -> ("Value"=w688:refnum<vi>)  [unwired: 2 in, 2 out]
                            n524 = property on="6485 Samples/measurement" class="LVObjRef (strict)"() -> ("Value"=w635:refnum<vi>)  [unwired: 2 in, 2 out]
                            n525 = property on="6487 Samples/measurement" class="LVObjRef (strict)"() -> ("Value"=w637:refnum<vi>)  [unwired: 2 in, 2 out]
                            n526 = property class="DigNum (strict)"(reference=w643) -> ("Value"=w667:dbl)  [unwired: 1 in, 2 out]
                            n527 = property class="DigNum (strict)"(reference=w642) -> ("Value"=w668:dbl)  [unwired: 1 in, 2 out]
                            n528 = property class="DigNum (strict)"(reference=w640) -> ("Value"=w669:dbl)  [unwired: 1 in, 2 out]
                            n529 = property class="DigNum (strict)"(reference=w639) -> ("Value"=w670:dbl)  [unwired: 1 in, 2 out]
                            n530 = property class="DigNum (strict)"(reference=w671) -> ("Value"=w672:dbl)  [unwired: 1 in, 2 out]
                            n531 = property class="DigNum (strict)"(reference=w673) -> ("Value"=w674:dbl)  [unwired: 1 in, 2 out]
                            n532 = property class="DigNum (strict)"(reference=w675) -> ("Value"=w676:dbl)  [unwired: 1 in, 2 out]
                            n533 = property class="DigNum (strict)"(reference=w677) -> ("Value"=w678:dbl)  [unwired: 1 in, 2 out]
                            n534 = property class="DigNum (strict)"(reference=w679) -> ("Value"=w680:dbl)  [unwired: 1 in, 2 out]
                            n535 = property class="DigNum (strict)"(reference=w682) -> ("Value"=w681:dbl)  [unwired: 1 in, 2 out]
                            n536 = property class="DigNum (strict)"(reference=w683) -> ("Value"=w684:dbl)  [unwired: 1 in, 2 out]
                            n537 = property class="DigNum (strict)"(reference=w685) -> ("Value"=w686:dbl)  [unwired: 1 in, 2 out]
                            n538 = property class="DigNum (strict)"(reference=w687) -> ("Value"=w690:dbl)  [unwired: 1 in, 2 out]
                            n539 = property class="DigNum (strict)"(reference=w688) -> ("Value"=w689:dbl)  [unwired: 1 in, 2 out]
                            n540 = property class="DigNum (strict)"(reference=w635) -> ("Value"=w636:i32)  [unwired: 1 in, 2 out]
                            n541 = property class="DigNum (strict)"(reference=w637) -> ("Value"=w644:i32)  [unwired: 1 in, 2 out]
                            n542 = property class="DigNum (strict)"(reference=w646) -> ("Value"=w645:dbl)  [unwired: 1 in, 2 out]
                            n543 = property on="Keithley6485 Current (A)" class="LVObjRef (strict)"() -> ("Value"=w641:refnum<vi>)  [unwired: 2 in, 2 out]
                            n544 = property on="Keithley6487 Current (A)" class="LVObjRef (strict)"() -> ("Value"=w638:refnum<vi>)  [unwired: 2 in, 2 out]
                            n545 = property on="GM2 Counts" class="LVObjRef (strict)"() -> ("Value"=w634:refnum<vi>)  [unwired: 2 in, 2 out]
                            n546 = property on="GM1 Counts" class="LVObjRef (strict)"() -> ("Value"=w633:refnum<vi>)  [unwired: 2 in, 2 out]
                            n547 = property class="DigNum (strict)"(reference=w634) -> ("Value"=w632:i32)  [unwired: 1 in, 2 out]
                            n548 = property class="DigNum (strict)"(reference=w633) -> ("Value"=w631:i32)  [unwired: 1 in, 2 out]
                            n549 = property class="DigNum (strict)"(reference=w641) -> ("Value"=w648:dbl)  [unwired: 1 in, 2 out]
                            n550 = property class="DigNum (strict)"(reference=w638) -> ("Value"=w647:dbl)  [unwired: 1 in, 2 out]
                            n551 = Number To Fractional String(number=w667) -> (F-format string=w649:string)  [unwired: 3 in]
                            n552 = Number To Fractional String(number=w668) -> (F-format string=w650:string)  [unwired: 3 in]
                            n553 = Number To Fractional String(number=w669) -> (F-format string=w651:string)  [unwired: 3 in]
                            n554 = Number To Fractional String(number=w670) -> (F-format string=w652:string)  [unwired: 3 in]
                            n555 = Number To Fractional String(number=w672) -> (F-format string=w653:string)  [unwired: 3 in]
                            n556 = Number To Fractional String(number=w674) -> (F-format string=w654:string)  [unwired: 3 in]
                            n557 = Number To Fractional String(number=w676) -> (F-format string=w655:string)  [unwired: 3 in]
                            n558 = Number To Fractional String(number=w678) -> (F-format string=w656:string)  [unwired: 3 in]
                            n559 = Number To Fractional String(number=w680) -> (F-format string=w657:string)  [unwired: 3 in]
                            n560 = Number To Fractional String(number=w681) -> (F-format string=w658:string)  [unwired: 3 in]
                            n561 = Number To Fractional String(number=w684) -> (F-format string=w659:string)  [unwired: 3 in]
                            n562 = Number To Fractional String(number=w686) -> (F-format string=w660:string)  [unwired: 3 in]
                            n563 = Number To Fractional String(number=w690) -> (F-format string=w661:string)  [unwired: 3 in]
                            n564 = Number To Fractional String(number=w689) -> (F-format string=w662:string)  [unwired: 3 in]
                            n565 = Number To Decimal String(number=w636) -> (decimal integer string=w663:string)  [unwired: 1 in]
                            n566 = Number To Decimal String(number=w644) -> (decimal integer string=w664:string)  [unwired: 1 in]
                            n567 = Number To Fractional String(number=w645) -> (F-format string=w665:string)  [unwired: 3 in]
                            n568 = Number To Fractional String(number=w631) -> (F-format string=w628:string)  [unwired: 3 in]
                            n569 = Number To Exponential String(number=w648) -> (E-format string=w629:string)  [unwired: 3 in]
                            n570 = Number To Exponential String(number=w647) -> (E-format string=w630:string)  [unwired: 3 in]
                            n571 = property on="Voltage Supply A" class="LVObjRef (strict)"() -> ("Value"=w604:refnum<vi>)  [unwired: 2 in, 2 out]
                            n572 = property on="Voltage Supply B" class="LVObjRef (strict)"() -> ("Value"=w603:refnum<vi>)  [unwired: 2 in, 2 out]
                            n573 = property on="GM1 Dwell" class="LVObjRef (strict)"() -> ("Value"=w615:refnum<vi>)  [unwired: 2 in, 2 out]
                            n574 = property on="GM2 Dwell" class="LVObjRef (strict)"() -> ("Value"=w626:refnum<vi>)  [unwired: 2 in, 2 out]
                            n575 = property on="GM2 LLD" class="LVObjRef (strict)"() -> ("Value"=w619:refnum<vi>)  [unwired: 2 in, 2 out]
                            n576 = property on="GM2 ULD" class="LVObjRef (strict)"() -> ("Value"=w618:refnum<vi>)  [unwired: 2 in, 2 out]
                            n577 = property on="GM1 LLD" class="LVObjRef (strict)"() -> ("Value"=w621:refnum<vi>)  [unwired: 2 in, 2 out]
                            n578 = property on="GM1 ULD" class="LVObjRef (strict)"() -> ("Value"=w612:refnum<vi>)  [unwired: 2 in, 2 out]
                            n579 = property class="DigNum (strict)"(reference=w603) -> ("Value"=w601:dbl)  [unwired: 1 in, 2 out]
                            n580 = property on="Current File" class="Path"() -> ("Value"=w691:path)  [unwired: 2 in, 2 out]
                            n581 = Number To Fractional String(number=w632) -> (F-format string=w627:string)  [unwired: 3 in]
                            n582 = property class="DigNum (strict)"(reference=w604) -> ("Value"=w602:dbl)  [unwired: 1 in, 2 out]
                            n583 = property class="DigNum (strict)"(reference=w626) -> ("Value"=w625:dbl)  [unwired: 1 in, 2 out]
                            n584 = property class="DigNum (strict)"(reference=w619) -> ("Value"=w623:dbl)  [unwired: 1 in, 2 out]
                            n585 = property class="DigNum (strict)"(reference=w618) -> ("Value"=w617:dbl)  [unwired: 1 in, 2 out]
                            n586 = property class="DigNum (strict)"(reference=w615) -> ("Value"=w614:dbl)  [unwired: 1 in, 2 out]
                            n587 = property class="DigNum (strict)"(reference=w621) -> ("Value"=w620:dbl)  [unwired: 1 in, 2 out]
                            n588 = property class="DigNum (strict)"(reference=w612) -> ("Value"=w611:dbl)  [unwired: 1 in, 2 out]
                            n589 = Number To Fractional String(number=w601) -> (F-format string=w599:string)  [unwired: 3 in]
                            n590 = Number To Fractional String(number=w602) -> (F-format string=w600:string)  [unwired: 3 in]
                            n591 = Number To Fractional String(number=w625) -> (F-format string=w624:string)  [unwired: 3 in]
                            n592 = Number To Fractional String(number=w623) -> (F-format string=w622:string)  [unwired: 3 in]
                            n593 = Number To Fractional String(number=w620) -> (F-format string=w610:string)  [unwired: 3 in]
                            n594 = Number To Fractional String(number=w611) -> (F-format string=w609:string)  [unwired: 3 in]
                            n595 = Number To Fractional String(number=w617) -> (F-format string=w616:string)  [unwired: 3 in]
                            n596 = Number To Fractional String(number=w614) -> (F-format string=w613:string)  [unwired: 3 in]
                            n597 = Build Array(w605, w649, w650, w651, w652, w653, w654, w655, w656, w657, w658, w659, w660, w661, w662, w663, w664, w665, w624, w622, w616, w613, w610, w609, w600, w599, w598) -> (w666:string[])
                            n598 = Build Array (concatenate)(w666, w627, w628, w629, w630) -> (w694:string[])
                            n599 = call-poly <vilib>:"Write To Spreadsheet File.vi"("format (%s)"="%e" ("format (%.3f)"), "append to file? (new file:F)"=TRUE, "1D data"=w694, "file path (dialog if empty)"=w691) -> ()  [unwired: 4 in, 1 out]
                          }
                        }
                      }
                      frame "end" {
                        n600 = property on="Run All" class="Bool (strict)"() -> ("Value"=w699:bool)  [unwired: 2 in, 2 out]
                        n601 = property on="Current Task" class="Arr (strict)"() -> ("Value"=w698:string[])  [unwired: 2 in, 2 out]
                        n602 = property on="Current Scan" class="Str"() -> ("Value"=w702:string)  [unwired: 2 in, 2 out]
                        n603 = case shown="False" w699 {
                          frame False {
                            n604 = property on="Scan in Progress" class="LVObjRef (strict)"() -> ("Value"=w705:refnum<vi>)  [unwired: 2 in, 2 out]
                            n605 = property class="Bool (strict)"(reference=w705, "Value"=FALSE ("Scan In Progress")) -> ()  [unwired: 1 in, 2 out]
                          }
                          frame True {
                          }
                        }
                        n606 = Concatenate Strings("~Finished~\n" ("string"), w702) -> (w701:string)
                        n607 = Delete From Array(array=w698, index=0) -> (array with subset deleted=w697:string[])  [unwired: 1 in, 1 out]
                        n608 = property on="Current Action" class="Str"("Value"="") -> ()  [unwired: 2 in, 2 out]
                        n609 = property on="Current Scan" class="Str"("Value"=w701) -> ()  [unwired: 2 in, 2 out]
                        n610 = property on="Current Task" class="Arr (strict)"("Value"=w697) -> ()  [unwired: 2 in, 2 out]
                        n611 = property on="Progress:" class="DigNum (strict)"("Value"=100 ("Progress:")) -> ()  [unwired: 2 in, 2 out]
                      }
                      frame "format" {
                        n612 = String Subset(string=w722, offset (0)=1) -> (substring=w707:string)  [unwired: 1 in]
                        n613 = property on="Current File" class="Path"() -> ("Value"=w719:path)  [unwired: 2 in, 2 out]
                        n614 = Equal?(x=w707, y="\\n") -> (x = y?=w708:bool)
                        n615 = property on="Current Task" class="Arr (strict)"() -> ("Value"=w710:string[])  [unwired: 2 in, 2 out]
                        n616 = case shown="False" w708 {
                          tunnel: w707 -> [w723 _]
                          tunnel: [w723 "\r\n"] -> w706
                          frame False {
                          }
                          frame True {
                          }
                        }
                        n617 = Delete From Array(array=w710, index=0) -> (deleted portion=w711:string, array with subset deleted=w709:string[])  [unwired: 1 in]
                        n618 = Open/Create/Replace File(file path (use dialog)=w719, operation (0:open)=T2."open", access (0:read/write)=enum16{"read/write", "read-only", "write-only"}."read/write") -> (refnum out=w716:refnum<file>)  [unwired: 3 in, 2 out]
                        n619 = property on="Current Action" class="Str"("Value"=w711) -> ()  [unwired: 2 in, 2 out]
                        n620 = property on="Current Task" class="Arr (strict)"("Value"=w709) -> ()  [unwired: 2 in, 2 out]
                        n621 = Set File Position(refnum=w716, from (0:start)=enum16{"start", "end", "current"}."end") -> (refnum out=w713:refnum<file>)  [unwired: 2 in, 1 out]
                        n622 = Write to Text File(file (use dialog)=w713, text=w706) -> (refnum out=w714:refnum<file>)  [unwired: 2 in, 2 out]
                        n623 = Close File(refnum=w714) -> ()  [unwired: 1 in, 2 out]
                      }
                      frame "error", Default {
                        n624 = property on="Status" class="Str"("Value"="An error has occurred" ("Status")) -> ()  [unwired: 2 in, 2 out]
                      }
                    }
                  }
                  frame #1 {
                    n625 = property on="Current Action" class="Str"() -> ("Value"=w811:string)  [unwired: 2 in, 2 out]
                    n626 = Not Equal?(x="", y=w811) -> (x != y?=w809:bool)
                    n627 = case shown="True" w809 {
                      frame False {
                      }
                      frame True {
                        # "Clean up."
                        n628 = property on="Current Action" class="Str"() -> ("Value"=w815:string)  [unwired: 2 in, 2 out]
                        n629 = property on="Current Task" class="Arr (strict)"() -> ("Value"=w812:string[])  [unwired: 2 in, 2 out]
                        n630 = Insert Into Array(array=w812, index=0, new element=w815) -> (w813:string[])
                        n631 = property on="Current Task" class="Arr (strict)"("Value"=w813) -> ()  [unwired: 2 in, 2 out]
                      }
                    }
                  }
                }
              }
              frame True {
                n632 = property on="Scan in Progress" class="LVObjRef (strict)"() -> ("Value"=w818:refnum<vi>)  [unwired: 2 in, 2 out]
                n633 = property class="Bool (strict)"(reference=w818, "Value"=FALSE ("Scan In Progress")) -> ()  [unwired: 1 in, 2 out]
                n634 = property on="Current Scan" class="Str"("Value"="Scan queue empty" ("Current Scan")) -> ()  [unwired: 2 in, 2 out]
                n635 = flat-sequence {
                  frame #0 {
                    n636 = call <vilib>:"Beep.vi"("use system alert? (T)"=FALSE, "duration (msec)"=u32 150, "frequency (Hz)"=u32 300) -> ()  [unwired: 9 in]
                  }
                  frame #1 {
                    n637 = call <vilib>:"Beep.vi"("use system alert? (T)"=FALSE, "duration (msec)"=u32 150, "frequency (Hz)"=u32 300 ("duration (msec)")) -> ()  [unwired: 9 in]
                  }
                  frame #2 {
                    n638 = call <vilib>:"Beep.vi"("use system alert? (T)"=FALSE, "duration (msec)"=u32 150, "frequency (Hz)"=u32 300 ("duration (msec)")) -> ()  [unwired: 9 in]
                  }
                }
                "Run All" <- FALSE ("Run All")
              }
            }
          }
        }
      }
    }
  }
